vi "Autonomous Independent.vi"() -> ()   [LabVIEW 2016]
doc: "This VI is called when autonomous begins, and will automatically be terminated when autonomous ends. You can carry out timed or sensor driven robot movement independently without needing to return to the caller."
uses:
  <vilib>/Rock Robotics/WPI/ThirdParty/CanMotor/TalonSRX/WPI_CANTalonSRX_APIFeedbackSelect.ctl
  <vilib>/Rock Robotics/WPI/ThirdParty/CanMotor/TalonSRX/WPI_CANTalonSRX_Params.ctl
  <vilib>/Rock Robotics/WPI/ThirdParty/CanMotor/TalonSRX/WPI_CANTalonSRX_APIControlMode.ctl
  <vilib>/Rock Robotics/WPI/Utilities/WPI_GetSetVariantRefNum.vi
  <vilib>/Rock Robotics/Network Tables/NT Read String.vi
  <vilib>/Rock Robotics/Network Tables/NT Write Numeric Array.vi
  <vilib>/Rock Robotics/WPI/RobotDrive/WPI_RobotDriveArcadeDrive_Standard(NoSaturation).vi
  Robot Global Data.vi
panel:
  out "Distance":dbl
  out "Current":dbl
  out "CURRENT":dbl
  out "Distance 5":dbl
  out "Distance 4":dbl
  out "Distance 3":dbl
  out "RIGHT SIDE":dbl
  out "Encoder Position 4":dbl
  out "Encoder Position 3":dbl
  out "Encoder Position":dbl
  out "Encoder Position 2":dbl
  # "Be sure to right-click and choose Data Operations>>Make Current Value default if you want to save the array values with the VI"
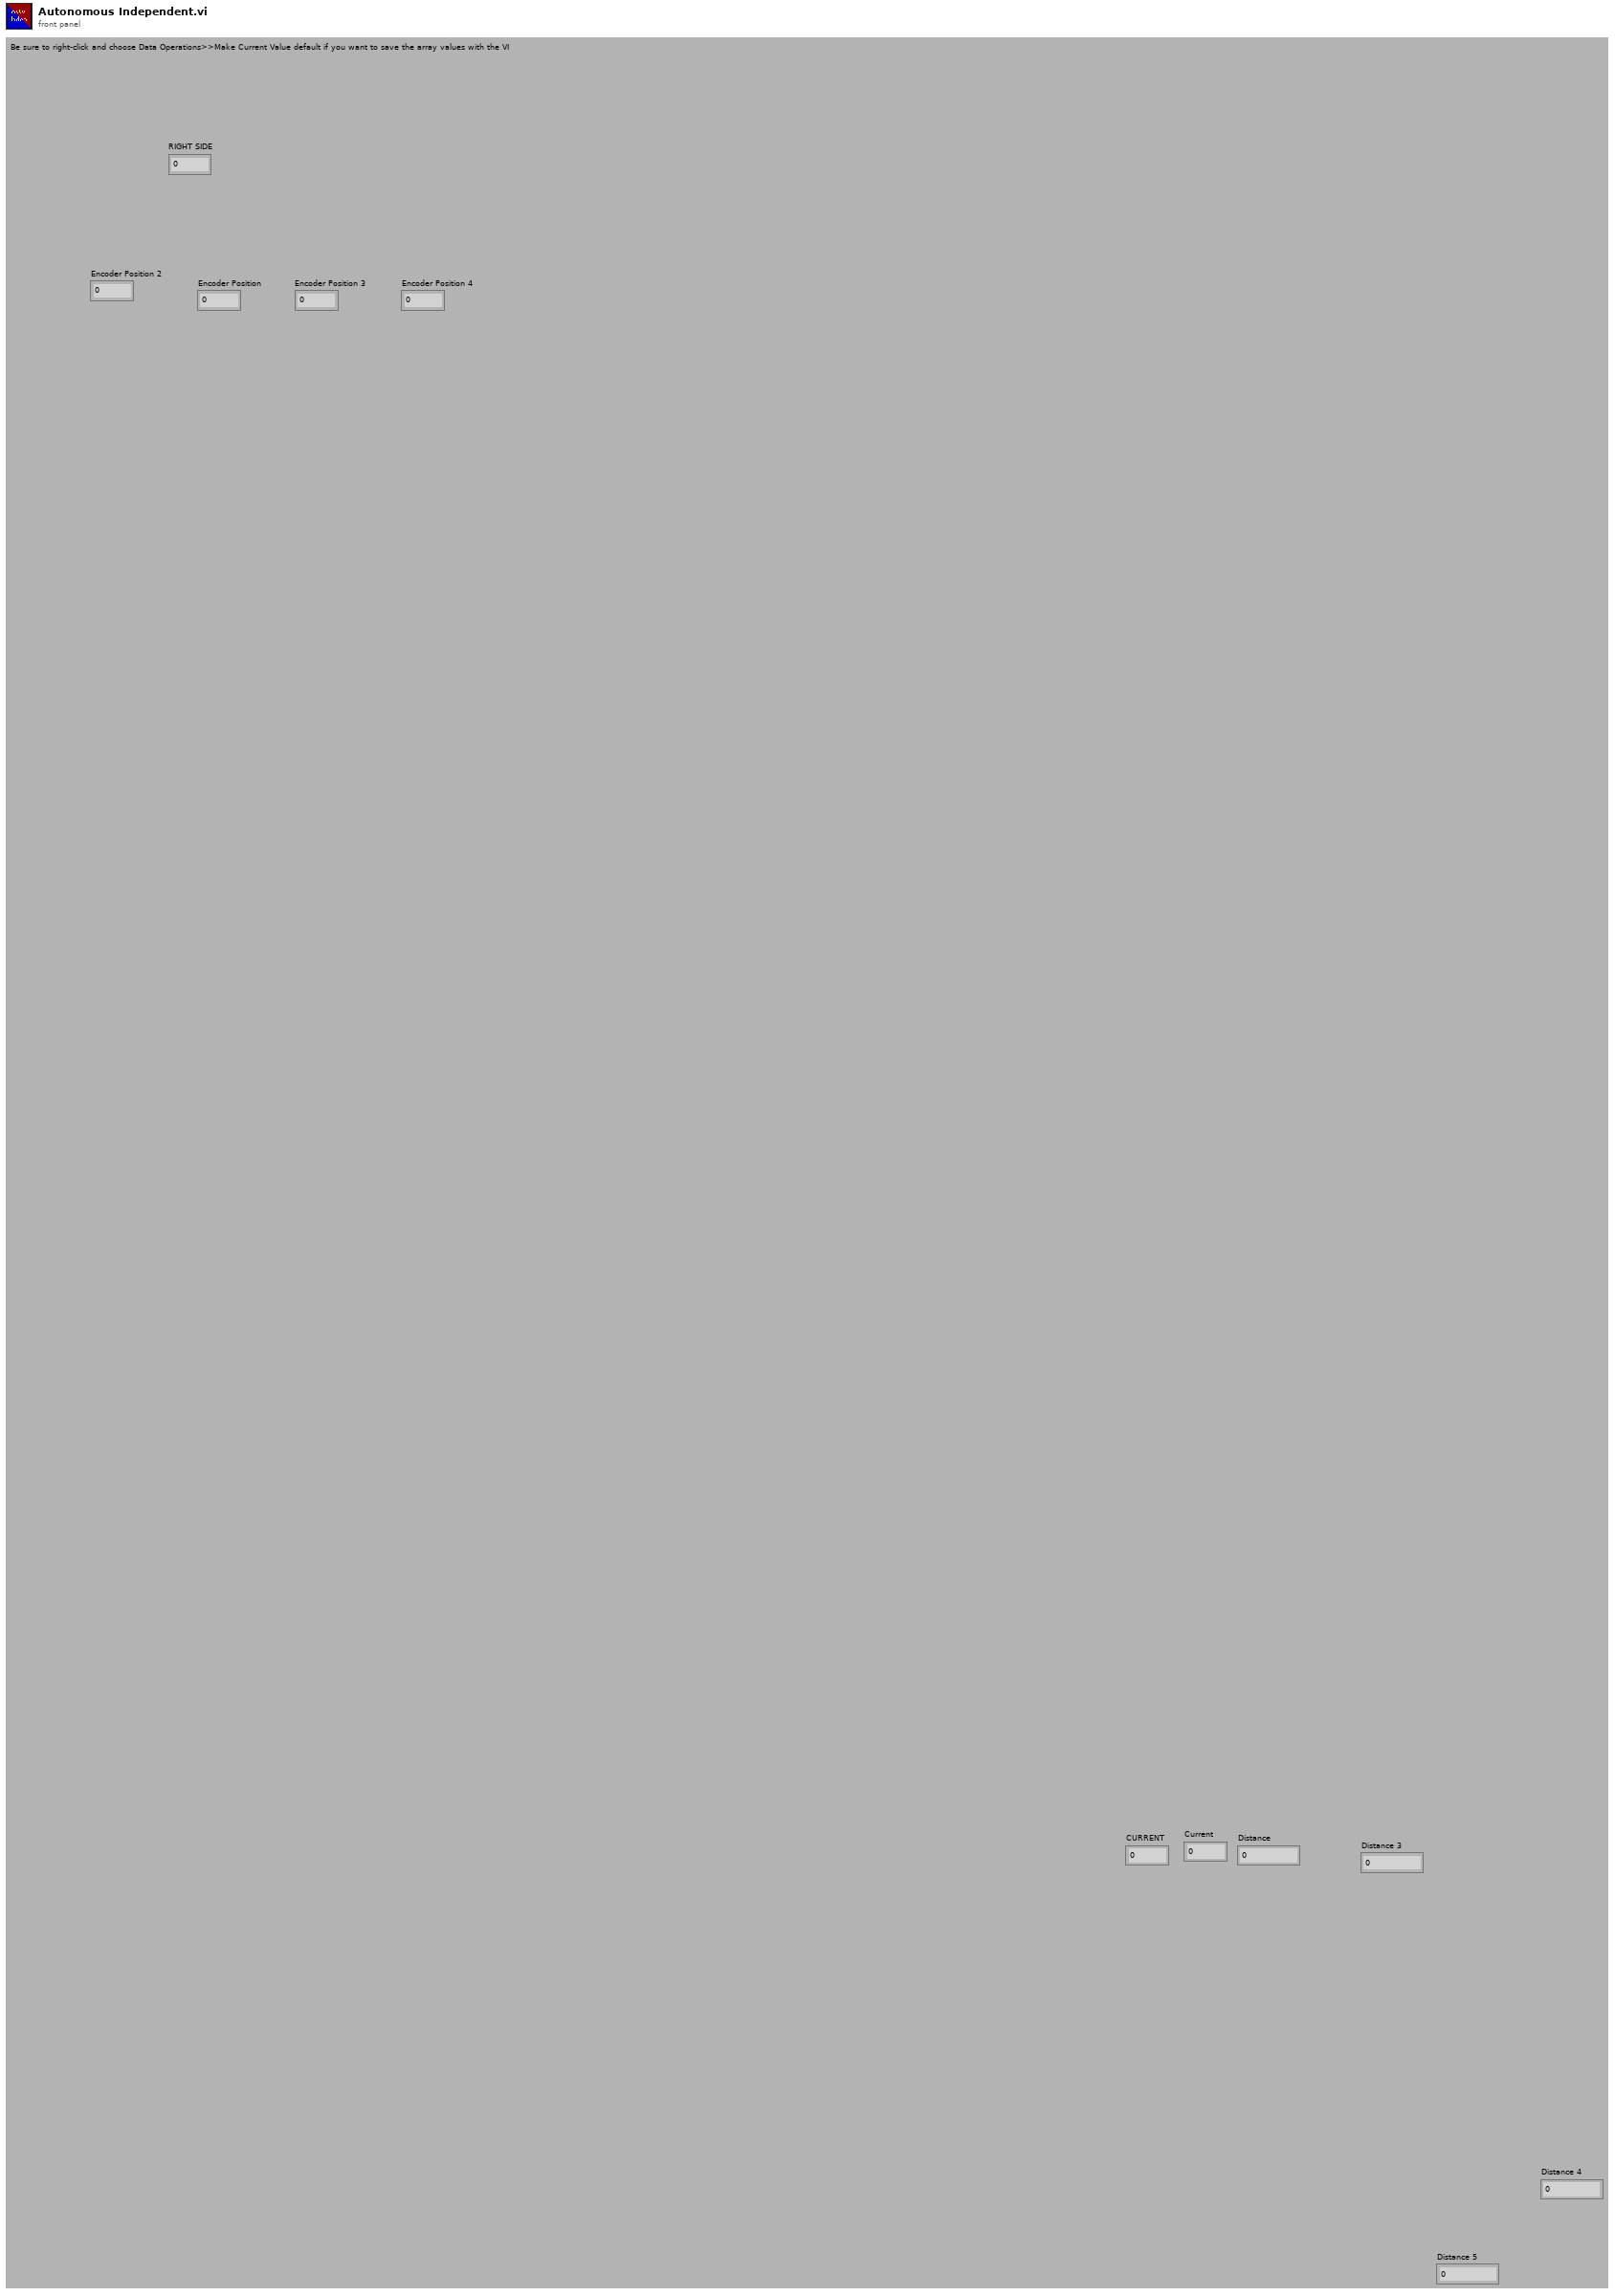
[diagram p1: front panel]
types:
  T1 = typedef "WPI_JoystickDevRef.ctl" = cluster{"Device":T2}
  T2 = typedef "WPI_JoystickDeviceEnum.ctl" = enum16{"USB 0", "USB 1", "USB 2", "USB 3", "USB 4", "USB 5"}
  T3 = typedef "WPI_EncoderDevRef.ctl" = cluster{"DevStatus":errorcluster, "EncoderIndex":T4, "CounterIndex":T5, "DistancePerCount":dbl, "Decoding Type":T6}
  T4 = typedef "FPGA_EncoderIdx.ctl" = enum8{"Enc 0", "Enc 1", "Enc 2", "Enc 3", "Enc 4", "Enc 5", "Enc 6", "Enc 7", "Invalid"}
  T5 = typedef "FPGA_CounterCtrSystemIndex.ctl" = enum8{"Ctr 0", "Ctr 1", "Ctr 2", "Ctr 3", "Ctr 4", "Ctr 5", "Ctr 6", "Ctr 7", "Invalid"}
  T6 = typedef "WPI_EncoderType.ctl" = enum16{"1x", "2x", "4x"}
  T7 = typedef "WPI_MotorControlDeviceRef.ctl" = cluster{"DeviceStatus":errorcluster, "Type":T8, "PWM":cluster{"PWM Channel":T9, "DeadBand":T10}, "CAN":cluster{"Device Number":u8, "SetOutput VI Ref":variant, "GetOutput VI Ref":variant, "Enable VI Ref":variant, "Disable VI Ref":variant, "Data":variant}, "Invert":bool}
  T8 = typedef "WPI_MotorControlType.ctl" = enum16{"PWM", "CAN"}
  T9 = typedef "FPGA_DIOPWMChannel.ctl" = enum8{"PWM 0", "PWM 1", "PWM 2", "PWM 3", "PWM 4", "PWM 5", "PWM 6", "PWM 7", "PWM 8", "PWM 9", "PWM MXP 0", "PWM MXP 1", "PWM MXP 2", "PWM MXP 3", "PWM MXP 4", "PWM MXP 5", "PWM MXP 6", "PWM MXP 7", "PWM MXP 8", "PWM MXP 9", "Invalid"}
  T10 = typedef "WPI_PWMDeadband.ctl" = cluster{"Name":string, "maxPositivePwm":i32, "minPositivePwm":i32, "centerPwm":i32, "maxNegativePwm":i32, "minNegativePwm":i32, "angularRange":u16}
  T11 = typedef "WPI_RobotDriveDevRef.ctl" = cluster{"DevStatus":errorcluster, "Motors[]":T7[], "Square Inputs":bool, "Max Output":dbl}
  T12 = typedef "WPI_CANTalonSRX_APIFeedbackSelect.ctl" = enum16{"Digital Quadrature Encoder", "Analog Potentiometer", "Analog Encoder", "Count on Quad-A (Rising-Edge)", "Count on Quad-A (Falling-Edge)", "CTR Magnetic Enc (Absolute)", "CTR Magnetic Enc (Relative)", "Pulse Width"}
  T13 = typedef "WPI_CANTalonSRX_APIControlMode.ctl" = enum8{"Percent VBus", "Speed", "Position", "Slave", "Unchanged / Invalid", "Voltage Compensation", "Current", "Motion Profile", "Motion Magic"}
  T14 = typedef "WPI_CANTalonSRX_Params.ctl" = u8
  T15 = typedef "WPI_CANTalonSRX_GlobalStatus.ctl" = cluster{"Applied Throttle":dbl, "Module Enabled":bool, "CAN Error":errorcluster, "Closed Loop Error":dbl, "Forward Limit Switch Closed":bool, "Reverse Limit Switch Closed":bool, "Sensor Position":dbl, "Sensor Velocity":dbl, "Current":dbl, "Sticky Fault - Over Temp":bool, "Sticky Fault - Under Voltage":bool, "Sticky Fault - Forward Limit":bool, "Sticky Fault - Reverse Limit":bool, "Sticky Fault - Forward Soft Limit":bool, "Sticky Fault - Reverse Soft Limit":bool, "Brake is Enabled":bool, "Encoder Position":dbl, "Encoder Velocity":dbl, "Encoder Index Count":dbl, "Encoder A Pin State":bool, "Encoder B Pin State":bool, "Encoder Index Pin State":bool, "Analog In":dbl, "Analog In Velocity":dbl, "Temperature (C)":dbl, "Battery Voltage":dbl, "Control 5 Is Supported":bool, "Current Profile Slot Select":dbl, "Pos Div 8":bool, "Vel Div 4":bool, "Pulse Width Position":i32, "Pulse Width Velocity":i32, "Pulse Width Rise To Rise (us)":i32, "Pulse Width Rise To Fall (us)":i32, "Mot Prof Active Is Under Run":bool, "Mot Prof Active Has Under Run":bool, "Mot Prof Active Is Last":bool, "Mot Prof Active Velocity Only":bool, "Mot Prof Active Is Valid":bool, "Mot Prof Buffer Is Full":bool, "Mot Prof Active Profile Slot Select":i32, "Mot Prof NextID":i32, "Mot Prof Count":i32, "Mot Prof Active Velocity":dbl, "Mot Prof Active Position":dbl, "Mot Prof Output Enable":i32, "UsageFrame":u32}
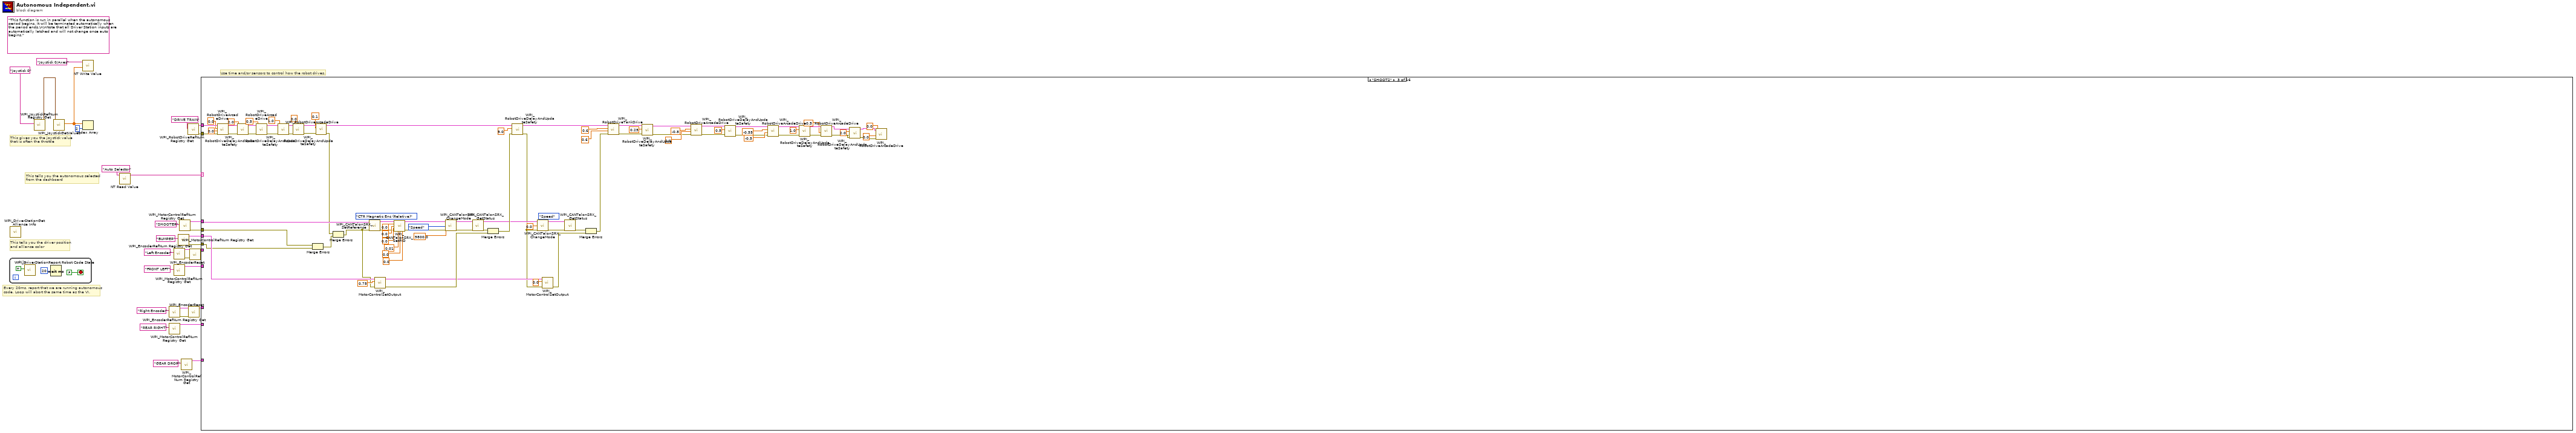
[diagram p0: block diagram]
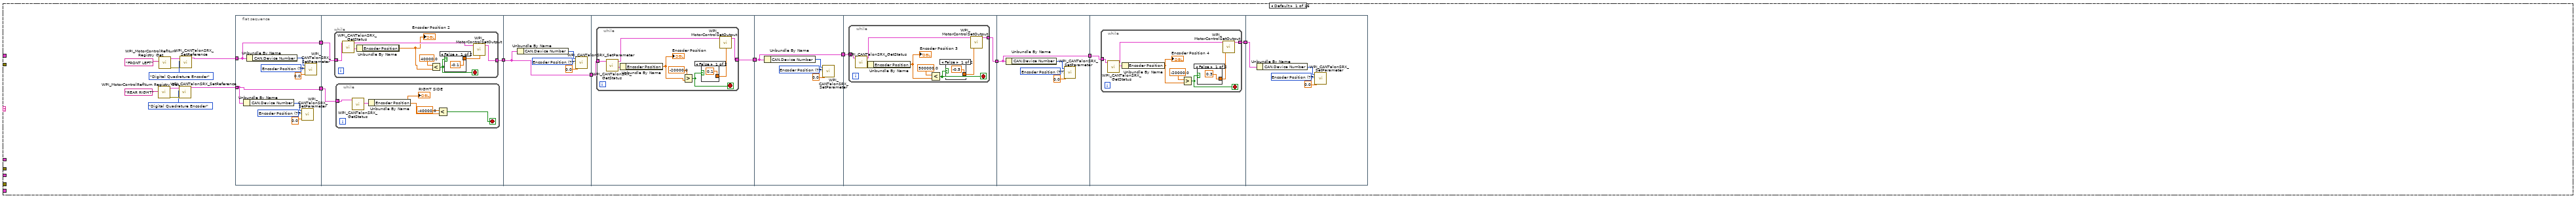
[diagram p2: hidden frame]
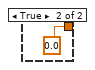
[diagram p3: hidden frame]
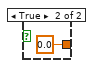
[diagram p4: hidden frame]
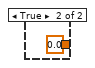
[diagram p5: hidden frame]
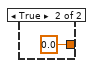
[diagram p6: hidden frame]
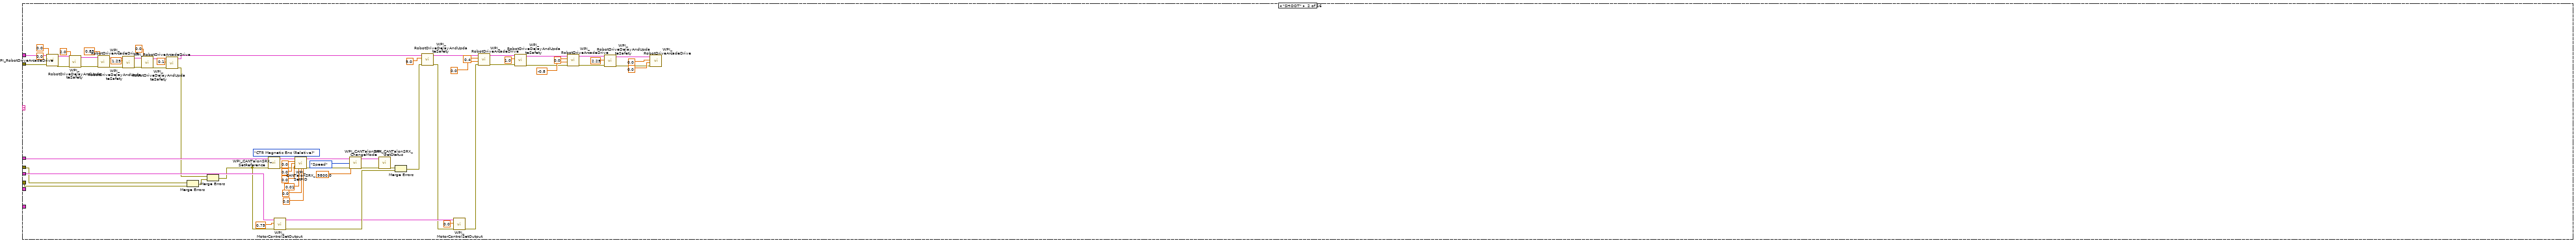
[diagram p7: hidden frame]
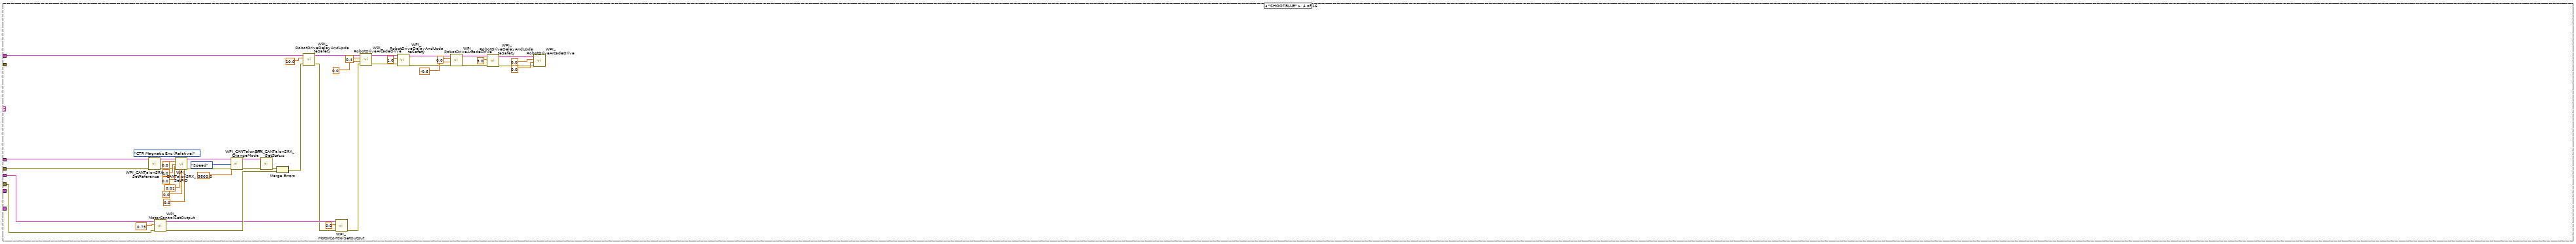
[diagram p8: hidden frame]
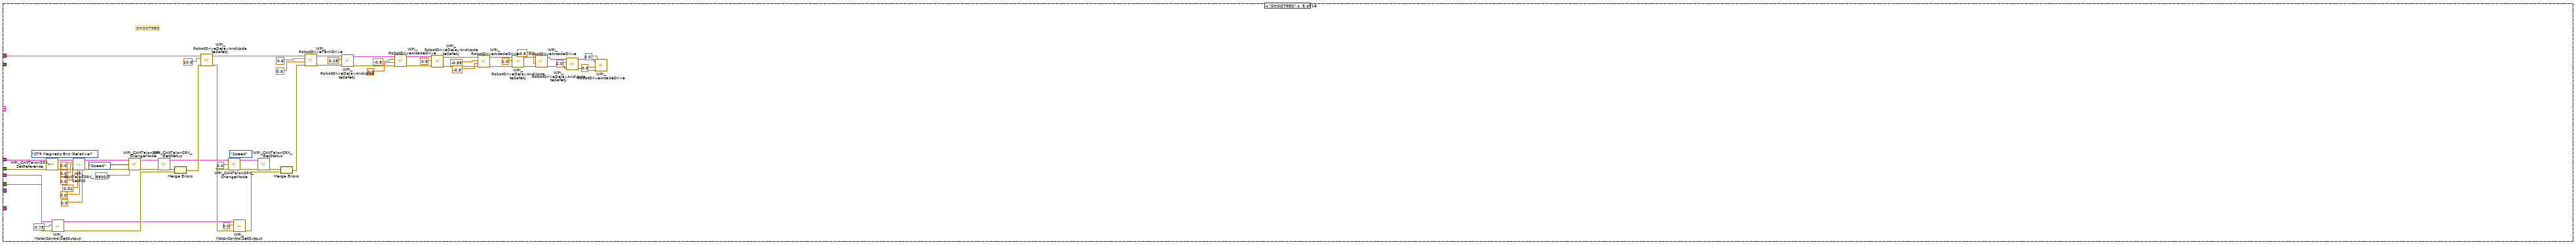
[diagram p9: hidden frame]
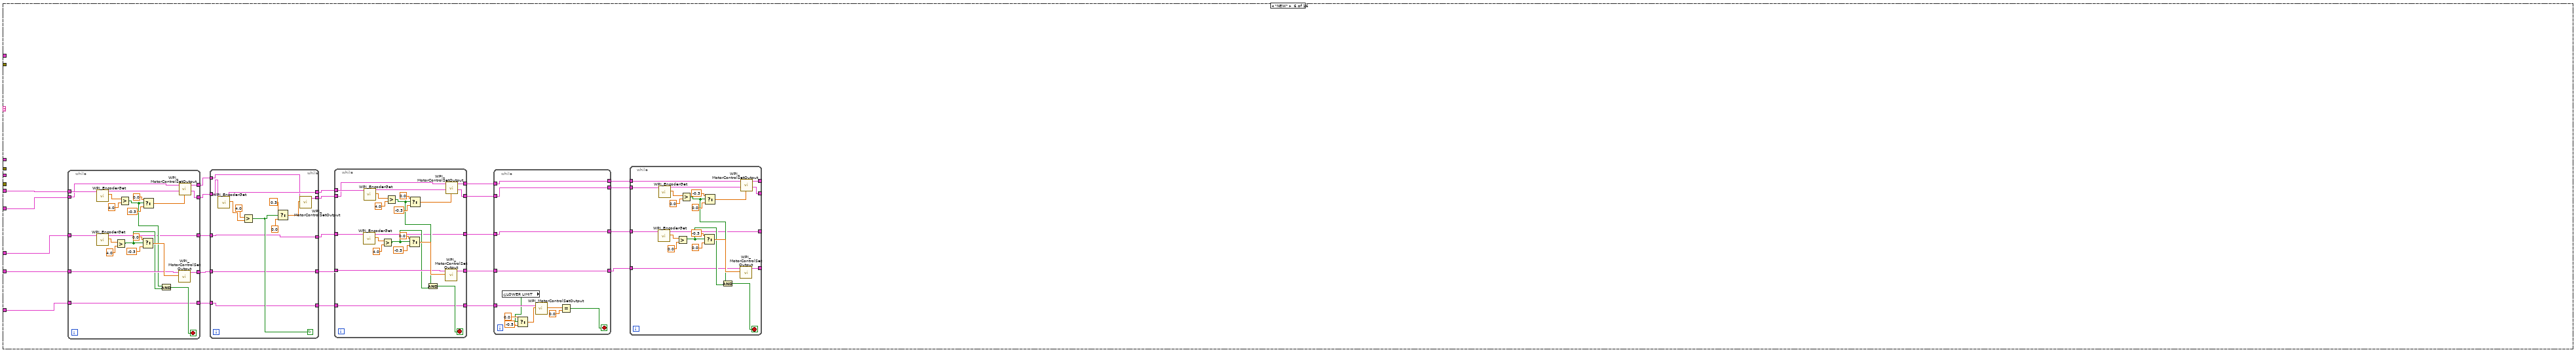
[diagram p10: hidden frame]
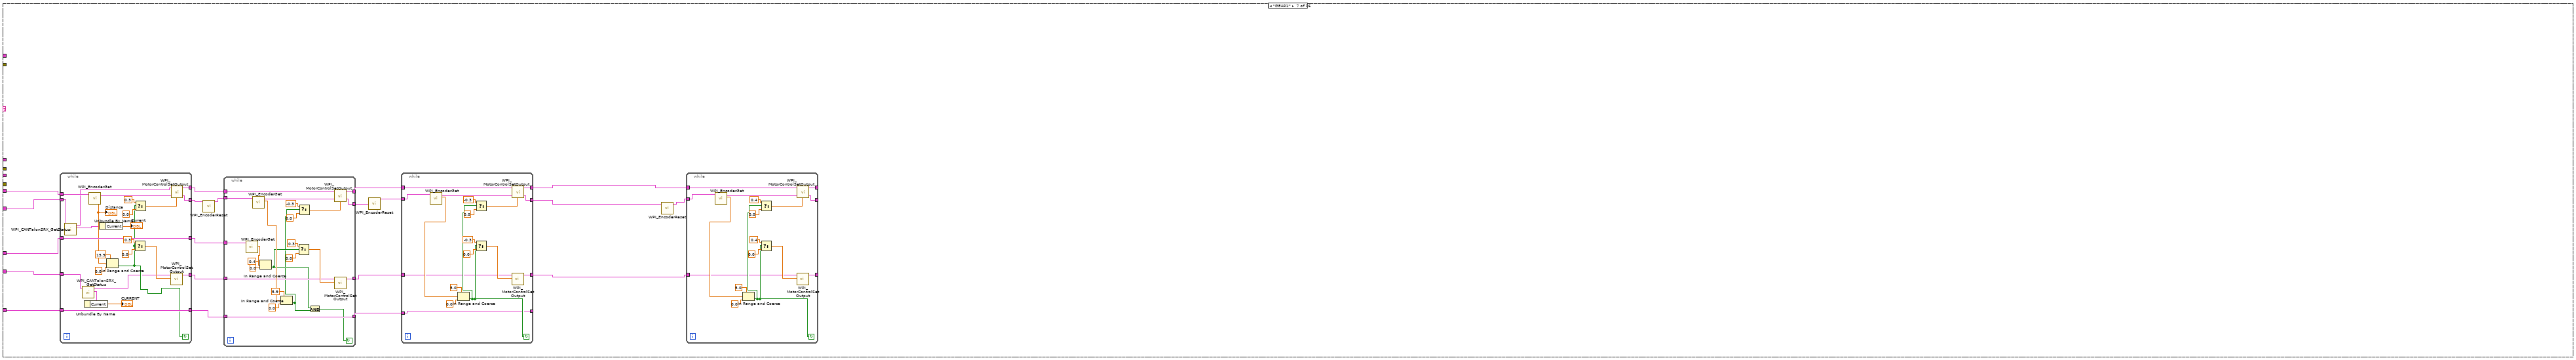
[diagram p11: hidden frame]
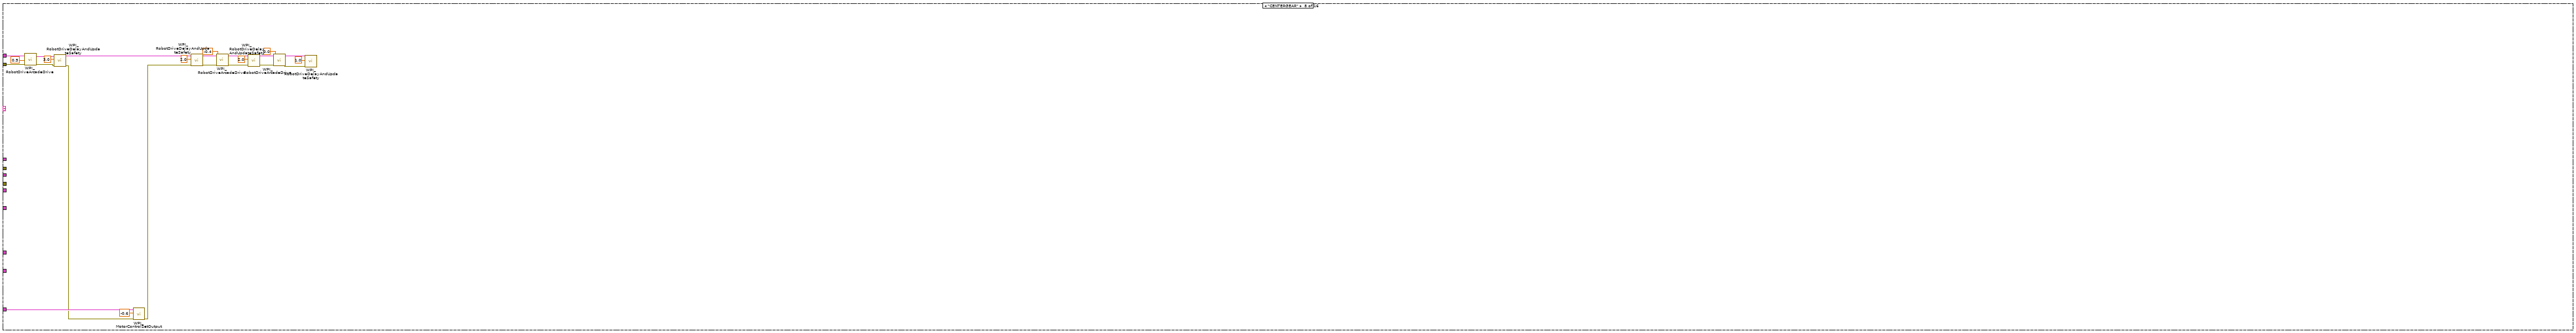
[diagram p12: hidden frame]
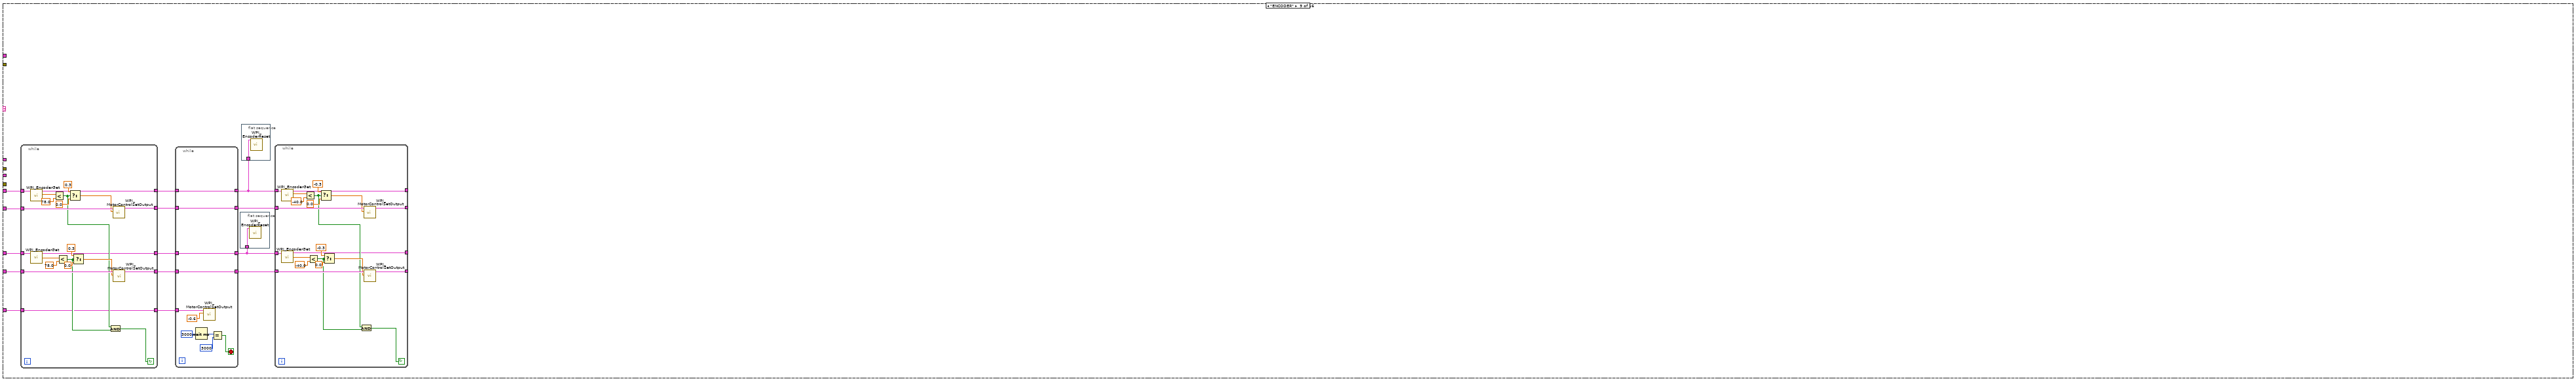
[diagram p13: hidden frame]
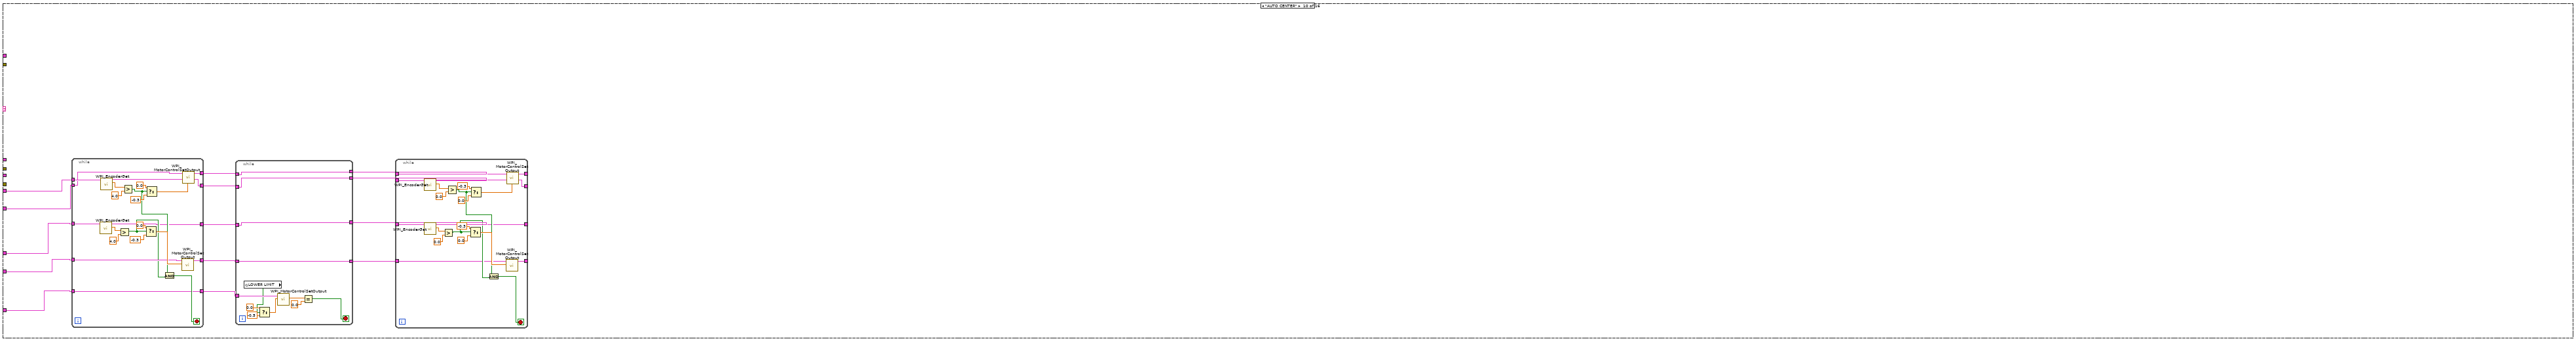
[diagram p14: hidden frame]
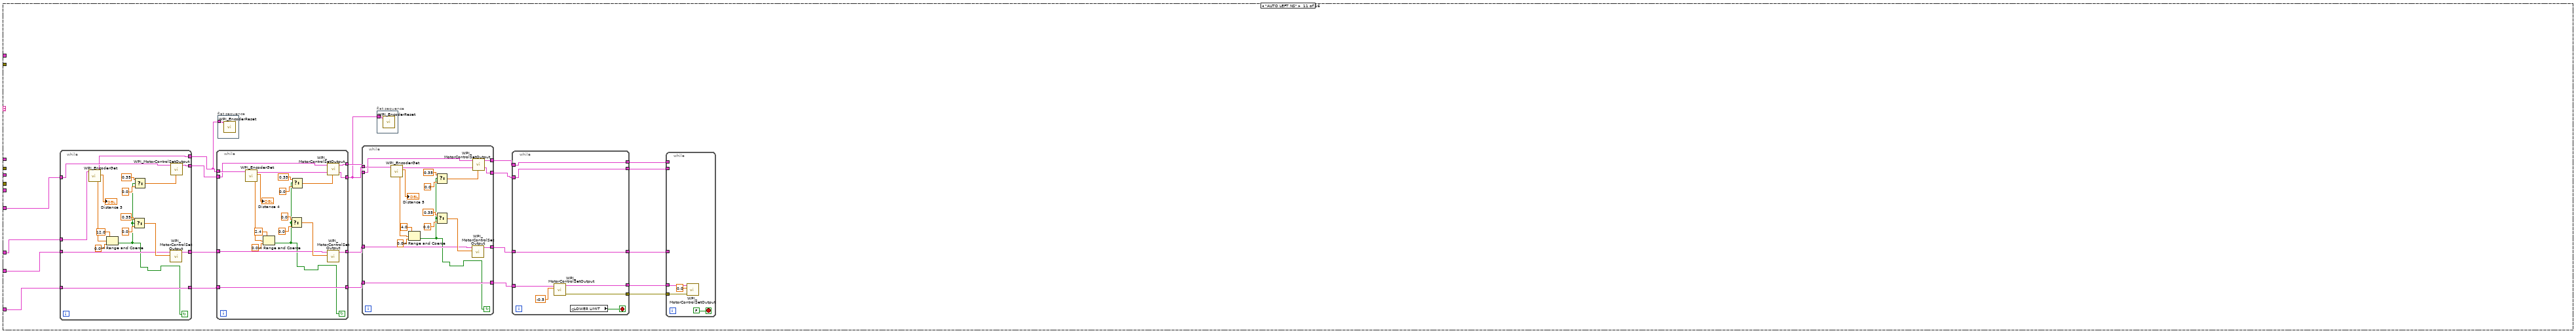
[diagram p15: hidden frame]
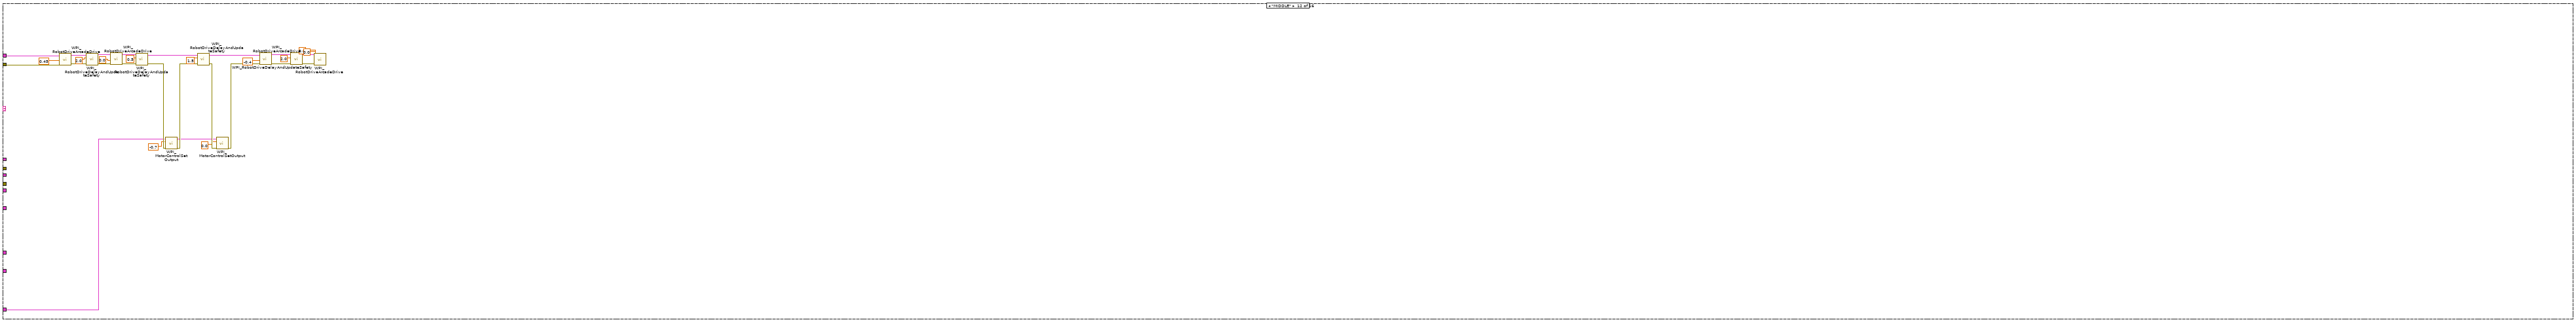
[diagram p16: hidden frame]
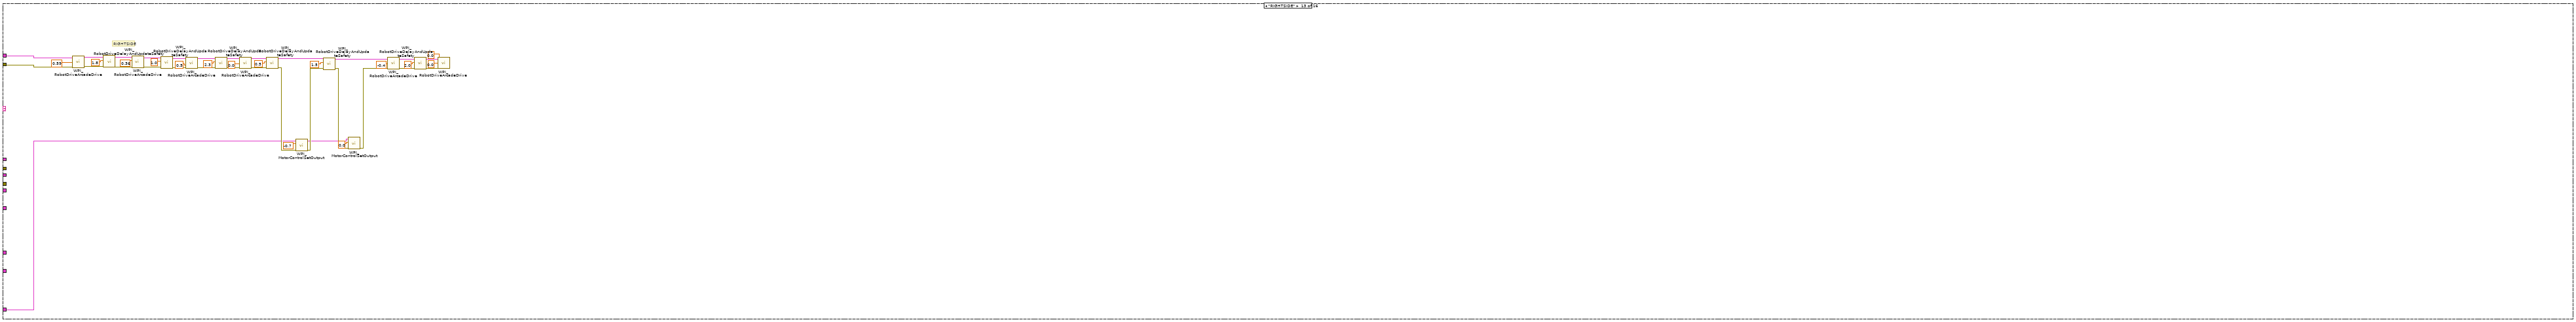
[diagram p17: hidden frame]
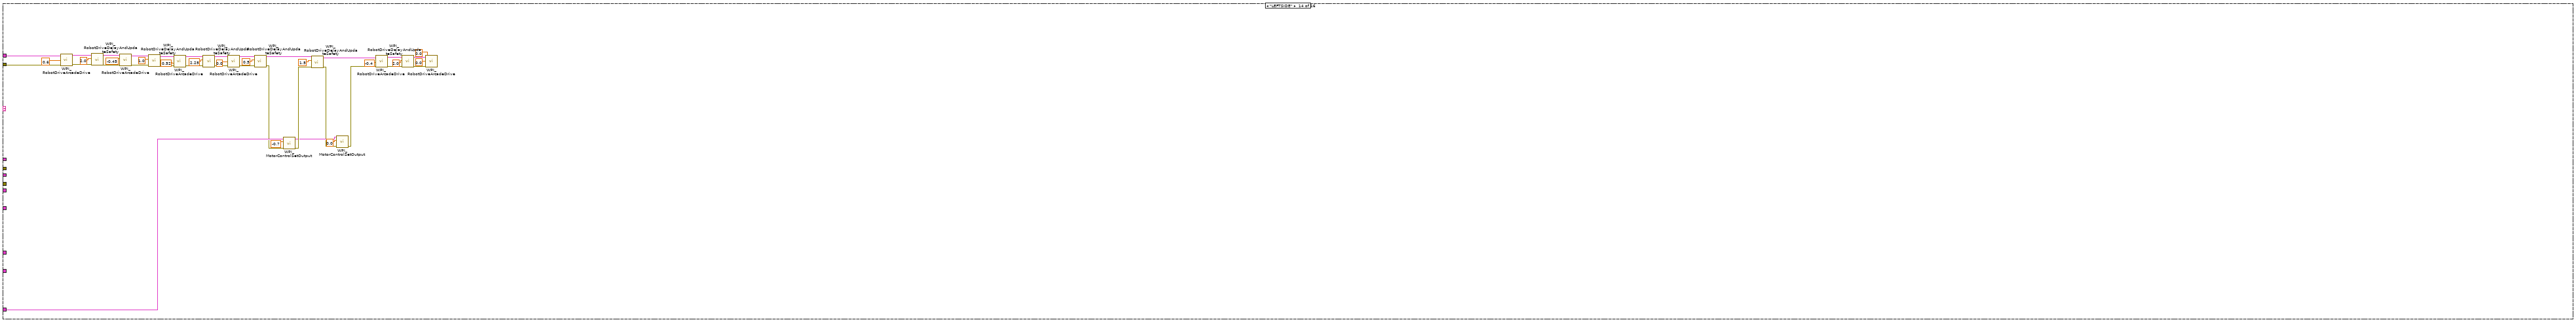
[diagram p18: hidden frame]
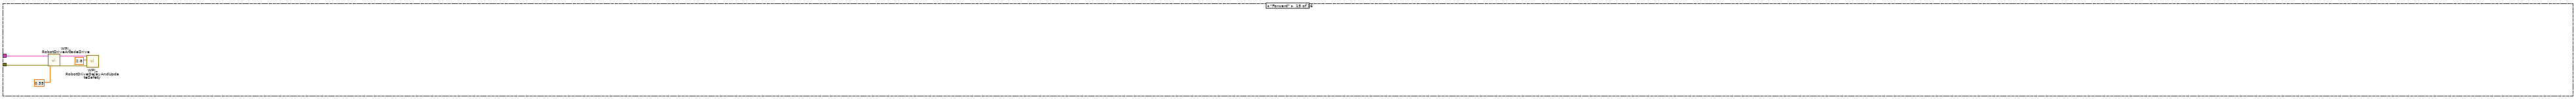
[diagram p19: hidden frame]
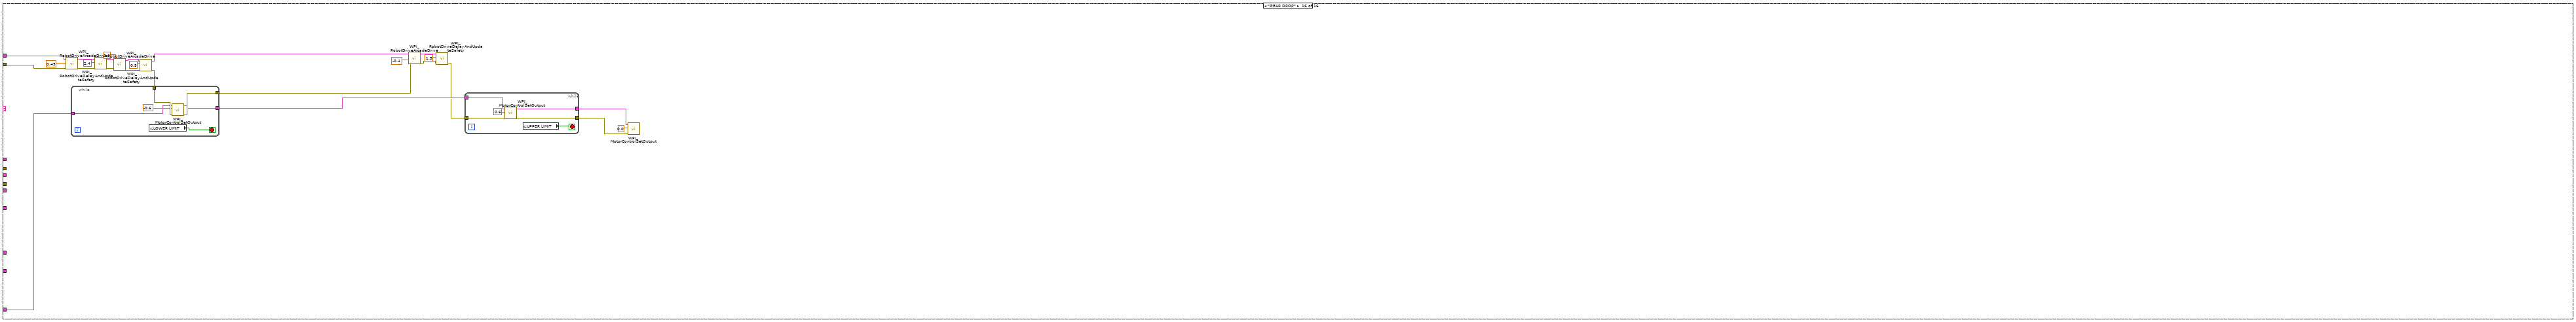
[diagram p20: hidden frame]
diagram:
  (unwired) "This function is run in parallel when the autonomous period begins. It will be terminated automatically when the period ends.\n\nNote that all Driver Station inputs are automatically latched and will not change once auto begins."
  # "Use time and/or sensors to control how the robot drives."
  # "This tells you the autonomous selected\nfrom the dashboard"
  # "Every 20ms, report that we are running autonomous\ncode. Loop will abort the same time as the VI."
  # "This gives you the joystick value\nthat is often the throttle"
  # "This tells you the driver position\nand alliance color"
  n1 = while {
    stop <- FALSE stop-if-true
    n2 = call <vilib>:"WPI_DriverStationReport Robot Code State.vi"("Autonomous"=TRUE) -> ()  [unwired: 10 in, 1 out]
    n3 = Wait (ms)(milliseconds to wait=u32 20) -> ()  [unwired: 1 out]
  }
  n4 = call <vilib>:"WPI_DriverStationGet Alliance Info.vi"() -> ()  [unwired: 12 out]
  n5 = call <vilib>:"WPI_JoystickRefNum Registry Get.vi"("refnum name"="Joystick 0") -> ("JoystickDevRef"=w29:T1)  [unwired: 1 in, 9 out]
  n6 = call <vilib>:"WPI_JoystickGetValues.vi"("JoystickDevRef"=w29) -> ("Axes"=w25:dbl[])  [unwired: 6 in, 4 out]
  n7 = call-poly <vilib>:"NT Write Value.vi"("Numeric Array"=w25, "Name"="Joystick 0/Axes") -> ()  [unwired: 9 in, 1 out]
  n8 = Index Array(array=w25, index=2) -> ()  [unwired: 1 out]
  n9 = call-poly <vilib>:"NT Read Value.vi"("Name"="Auto Selector") -> ("String"=w26:string)  [unwired: 9 in, 1 out]
  n10 = call <vilib>:"WPI_EncoderRefNum Registry Get.vi"("refnum name"="Right Encoder") -> ("error out"=w6:errorcluster, "EncoderDevRef"=w5:T3)  [unwired: 9 in]
  n11 = call <vilib>:"WPI_MotorControlRefNum Registry Get.vi"("refnum name"="REAR RIGHT") -> ("MotorControlDevRef"=w7:T7)  [unwired: 9 in, 1 out]
  n12 = call <vilib>:"WPI_EncoderRefNum Registry Get.vi"("refnum name"="Left Encoder") -> ("error out"=w3:errorcluster, "EncoderDevRef"=w2:T3)  [unwired: 9 in]
  n13 = call <vilib>:"WPI_MotorControlRefNum Registry Get.vi"("refnum name"="FRONT LEFT") -> ("MotorControlDevRef"=w10:T7)  [unwired: 9 in, 1 out]
  n14 = call <vilib>:"WPI_MotorControlRefNum Registry Get.vi"("refnum name"="BUMPER") -> ("error out"=w14:errorcluster, "MotorControlDevRef"=w15:T7)  [unwired: 9 in]
  n15 = call <vilib>:"WPI_MotorControlRefNum Registry Get.vi"("refnum name"="SHOOTER") -> ("error out"=w16:errorcluster, "MotorControlDevRef"=w17:T7)  [unwired: 9 in]
  n16 = call <vilib>:"WPI_MotorControlRefNum Registry Get.vi"("refnum name"="GEAR DROP") -> ("MotorControlDevRef"=w19:T7)  [unwired: 9 in, 1 out]
  n17 = call <vilib>:"WPI_RobotDriveRefNum Registry Get.vi"("refnum name"="DRIVE TRAIN") -> ("error out"=w21:errorcluster, "RobotDriveDevRef"=w22:T11)  [unwired: 9 in]
  n18 = call <vilib>:"WPI_EncoderReset.vi"("error in (no error)"=w6, "EncoderDevRef"=w5) -> ("EncoderDevRef"=w4:T3)  [unwired: 8 in, 1 out]
  n19 = call <vilib>:"WPI_EncoderReset.vi"("error in (no error)"=w3, "EncoderDevRef"=w2) -> ("EncoderDevRef"=w1:T3)  [unwired: 8 in, 1 out]
  n20 = case shown="\"SHOOT2\"" w26 {
    tunnel: w22 -> [_ w156 w224 w291 w380 _ _ w636 _ _ _ w891 w894 w977 w983 w1008]
    tunnel: w21 -> [_ w155 w225 _ _ _ _ w635 _ _ _ w890 w893 w976 w982 w1007]
    tunnel: w19 -> [_ _ _ _ _ w406 w528 w630 w646 w715 w793 w878 w892 w953 _ w988]
    tunnel: w17 -> [_ w186 w205 w287 w386 _ _ _ _ _ _ _ _ _ _ _]
    tunnel: w16 -> [_ w143 w203 w288 w385 _ _ _ _ _ _ _ _ _ _ _]
    tunnel: w15 -> [_ w173 w204 w290 w373 _ _ _ _ _ _ _ _ _ _ _]
    tunnel: w14 -> [_ w142 w202 w289 w372 _ _ _ _ _ _ _ _ _ _ _]
    tunnel: w1 -> [_ _ _ _ _ w420 w531 _ w650 w719 _ _ _ _ _ _]
    tunnel: w10 -> [_ _ _ _ _ w419 w532 _ w649 w718 w795 _ _ _ _ _]
    tunnel: w7 -> [_ _ _ _ _ w417 w529 _ w647 w716 w794 _ _ _ _ _]
    tunnel: w4 -> [_ _ _ _ _ w418 w530 _ w648 w717 w775 _ _ _ _ _]
    frame Default {
      n21 = call <vilib>:"WPI_MotorControlRefNum Registry Get.vi"("refnum name"="REAR RIGHT") -> ("error out"=w38:errorcluster, "MotorControlDevRef"=w37:T7)  [unwired: 9 in]
      n22 = call <vilib>:"WPI_MotorControlRefNum Registry Get.vi"("refnum name"="FRONT LEFT") -> ("error out"=w50:errorcluster, "MotorControlDevRef"=w51:T7)  [unwired: 9 in]
      n23 = call <vilib>:"WPI_CANTalonSRX_SetReference.vi"("error in (no error)"=w38, "Feedback Reference"=WPI_CANTalonSRX_APIFeedbackSelect."Digital Quadrature Encoder", "CAN Talon SRX Ref"=w37) -> ("CAN Talon SRX Ref"=w35:T7)  [unwired: 7 in, 1 out]
      n24 = call <vilib>:"WPI_CANTalonSRX_SetReference.vi"("error in (no error)"=w50, "Feedback Reference"=WPI_CANTalonSRX_APIFeedbackSelect."Digital Quadrature Encoder", "CAN Talon SRX Ref"=w51) -> ("CAN Talon SRX Ref"=w46:T7)  [unwired: 7 in, 1 out]
      n25 = flat-sequence {
        tunnel: w46 -> [w57]
        tunnel: [w57] -> w45
        tunnel: w35 -> [w53]
        tunnel: [w53] -> w34
        tunnel: [w62] -> w48
        tunnel: w45 -> [w63]
        tunnel: w34 -> [w61]
        tunnel: w48 -> [w79]
        tunnel: [w79] -> w47
        tunnel: w47 -> [w84]
        tunnel: [w83] -> w44
        tunnel: w44 -> [w95]
        tunnel: [w95] -> w43
        tunnel: w43 -> [w100]
        tunnel: [w99] -> w42
        tunnel: w42 -> [w111]
        tunnel: [w111] -> w41
        tunnel: w41 -> [w116]
        tunnel: [w115] -> w40
        tunnel: w40 -> [w127]
        frame #0 {
          w55 = T14 77 items=["Slot 0 - P"=1, "Slot 0 - I"=2, "Slot 0 - D"=3, "Slot 0 - F"=4, "Slot 0 - I Zone"=5, "Slot 0 - Ramp Rate"=6, "Slot 1 - P"=11, "Slot 1 - I"=12, "Slot 1 - D"=13, "Slot 1 - F"=14, "Slot 1 - I Zone"=15, "Slot 1 - Ramp Rate"=16, "Soft Limit - Forward"=21, "Soft Limit - Reverse"=22, "Soft Limit - Forward Enable"=23, "Soft Limit - Reverse Enable"=24, "On Boot - Brake Mode"=31, "On Boot - Limit Normally Closed - Forward"=32, "On Boot - Limit Normally Closed - Reverse"=33, "On Boot - Limit Disabled - Forward"=34, "On Boot - Limit Disabled - Reverse"=35, "Fault - Over Temp"=41, "Fault - Under Voltage"=42, "Fault - Forward Limit"=43, "Fault - Reverse Limit"=44, "Fault - Hardware Failure"=45, "Fault - Forward Soft Limit"=46, "Fault - Reverse Soft Limit"=47, "Sticky Fault - Over Temp"=48, "Sticky Fault - Under Voltage"=49, "Sticky Fault - Forward Limit"=50, "Sticky Fault - Reverse Limit"=51, "Sticky Fault - Forward Soft Limit"=52, "Sticky Fault - Reverse Soft Limit"=53, "Applied Throttle"=61, "Closed-Loop Error"=62, "Select Feedback Device"=63, "Reverse Closed-Loop Output"=64, "Mode Select"=65, "Profile Slot Select"=66, "Ramp Throttle"=67, "Reverse Feedback Sensor"=68, "Limit Switch Enabled"=69, "Limit Switch Closed - Forward"=70, "Limit Switch Closed - Reverse"=71, "Sensor Position"=73, "Sensor Velocity"=74, "Current"=75, "Brake is Enabled"=76, "Encoder Position"=77, "Encoder Velocity"=78, "Encoder Index Rise Events"=79, "Encoder A Pin State"=80, "Encoder B Pin State"=81, "Encoder Index Pin State"=82, "Analog In with Overflow"=83, "Analog In Velocity"=84, "Temperature"=85, "Battery Voltage"=86, "Reset Count"=87, "Reset Flags"=88, "Firmware Version"=89, "Settings Changed"=90, "Quad Filter Enable"=91, "Ignore Disable Broadcast"=92, "I Accumulator"=93, "Status 1 Frame Rate Ms"=94, "Status 2 Frame Rate Ms"=95, "Status 3 Frame Rate Ms"=96, "Status 4 Frame Rate Ms"=97, "Status 6 Frame Rate Ms"=98, "Status 7 Frame Rate Ms"=99, "Enable Index Pin Clear Position"=100, "Peak Positive Output"=104, "Nominal Positive Output"=105, "Peak Negative Output"=106, "Nominal Negative Output"=107, "Quad Index Pin Polarity"=108, "Status 8 Frame Rate Ms"=109, "Allow Position Overflow"=110, "Slot 0 - Allowable Closed-Loop Error"=111, "Number Potentiometer Turns"=112, "Encoder Codes Per Rev"=113, "Pulse Width Decoded Position"=114, "Analog Position"=115, "Voltage Compensation Rate (V/s)"=116, "Slot 1 - Allowable Closed-Loop Error"=117, "Motion Profile Has Underrun Err"=119, "Reserved 120"=120, "Legacy Control Mode"=121, "Motion Magic Acceleration"=122, "Motion Magic Cruise Velocity"=123, "Status 10 Frame Rate"=124, "Current Limit Threshold"=125, "CustomParam0"=137, "CustomParam1"=138, "PersStorageSaving"=139, "ClearPositionOnLimitF"=144, "ClearPositionOnLimitR"=145, "NominalBatteryVoltage"=146, "SampleVelocityPeriod"=147, "SampleVelocityWindow"=148] ("Parameter")
          w59 = T14 77 items=["Slot 0 - P"=1, "Slot 0 - I"=2, "Slot 0 - D"=3, "Slot 0 - F"=4, "Slot 0 - I Zone"=5, "Slot 0 - Ramp Rate"=6, "Slot 1 - P"=11, "Slot 1 - I"=12, "Slot 1 - D"=13, "Slot 1 - F"=14, "Slot 1 - I Zone"=15, "Slot 1 - Ramp Rate"=16, "Soft Limit - Forward"=21, "Soft Limit - Reverse"=22, "Soft Limit - Forward Enable"=23, "Soft Limit - Reverse Enable"=24, "On Boot - Brake Mode"=31, "On Boot - Limit Normally Closed - Forward"=32, "On Boot - Limit Normally Closed - Reverse"=33, "On Boot - Limit Disabled - Forward"=34, "On Boot - Limit Disabled - Reverse"=35, "Fault - Over Temp"=41, "Fault - Under Voltage"=42, "Fault - Forward Limit"=43, "Fault - Reverse Limit"=44, "Fault - Hardware Failure"=45, "Fault - Forward Soft Limit"=46, "Fault - Reverse Soft Limit"=47, "Sticky Fault - Over Temp"=48, "Sticky Fault - Under Voltage"=49, "Sticky Fault - Forward Limit"=50, "Sticky Fault - Reverse Limit"=51, "Sticky Fault - Forward Soft Limit"=52, "Sticky Fault - Reverse Soft Limit"=53, "Applied Throttle"=61, "Closed-Loop Error"=62, "Select Feedback Device"=63, "Reverse Closed-Loop Output"=64, "Mode Select"=65, "Profile Slot Select"=66, "Ramp Throttle"=67, "Reverse Feedback Sensor"=68, "Limit Switch Enabled"=69, "Limit Switch Closed - Forward"=70, "Limit Switch Closed - Reverse"=71, "Sensor Position"=73, "Sensor Velocity"=74, "Current"=75, "Brake is Enabled"=76, "Encoder Position"=77, "Encoder Velocity"=78, "Encoder Index Rise Events"=79, "Encoder A Pin State"=80, "Encoder B Pin State"=81, "Encoder Index Pin State"=82, "Analog In with Overflow"=83, "Analog In Velocity"=84, "Temperature"=85, "Battery Voltage"=86, "Reset Count"=87, "Reset Flags"=88, "Firmware Version"=89, "Settings Changed"=90, "Quad Filter Enable"=91, "Ignore Disable Broadcast"=92, "I Accumulator"=93, "Status 1 Frame Rate Ms"=94, "Status 2 Frame Rate Ms"=95, "Status 3 Frame Rate Ms"=96, "Status 4 Frame Rate Ms"=97, "Status 6 Frame Rate Ms"=98, "Status 7 Frame Rate Ms"=99, "Enable Index Pin Clear Position"=100, "Peak Positive Output"=104, "Nominal Positive Output"=105, "Peak Negative Output"=106, "Nominal Negative Output"=107, "Quad Index Pin Polarity"=108, "Status 8 Frame Rate Ms"=109, "Allow Position Overflow"=110, "Slot 0 - Allowable Closed-Loop Error"=111, "Number Potentiometer Turns"=112, "Encoder Codes Per Rev"=113, "Pulse Width Decoded Position"=114, "Analog Position"=115, "Voltage Compensation Rate (V/s)"=116, "Slot 1 - Allowable Closed-Loop Error"=117, "Motion Profile Has Underrun Err"=119, "Reserved 120"=120, "Legacy Control Mode"=121, "Motion Magic Acceleration"=122, "Motion Magic Cruise Velocity"=123, "Status 10 Frame Rate"=124, "Current Limit Threshold"=125, "CustomParam0"=137, "CustomParam1"=138, "PersStorageSaving"=139, "ClearPositionOnLimitF"=144, "ClearPositionOnLimitR"=145, "NominalBatteryVoltage"=146, "SampleVelocityPeriod"=147, "SampleVelocityWindow"=148] ("Parameter")
          n26 = Unbundle By Name(w53) -> ("CAN.Device Number"=w54:u8)
          n27 = Unbundle By Name(w57) -> ("CAN.Device Number"=w60:u8)
          n28 = call <vilib>:"WPI_CANTalonSRX_SetParameter.vi"("Value"=0.0, "Parameter"=w55, "Device ID (0)"=w54) -> ()  [unwired: 7 in, 2 out]
          n29 = call <vilib>:"WPI_CANTalonSRX_SetParameter.vi"("Value"=0.0, "Parameter"=w59, "Device ID (0)"=w60) -> ()  [unwired: 7 in, 2 out]
        }
        frame #1 {
          n30 = while {
            tunnel: w63 -> [w70]
            tunnel: [w69] -> w62
            stop <- w73 stop-if-true
            n31 = call <vilib>:"WPI_CANTalonSRX_GetStatus.vi"("CAN Talon SRX Ref"=w70) -> ("Talon SRX Status"=w76:T15, "CAN Talon SRX Ref"=w75:T7)  [unwired: 8 in, 1 out]
            n32 = Unbundle By Name(w76) -> ("Encoder Position"=w72:dbl)
            "Encoder Position 2" <- w72
            n33 = Less?(x=40000.0, y=w72) -> (x < y?=w73:bool)
            n34 = case shown="False" w73 {
              tunnel: [-0.1 ("x") 0.0 ("x")] -> w74
              frame False {
              }
              frame True {
              }
            }
            n35 = call <vilib>:"WPI_MotorControlSetOutput.vi"("Output"=w74, "MotorControlDevRef"=w75) -> ("MotorControlDevRef"=w69:T7)  [unwired: 7 in, 2 out]
          }
          n36 = while {
            tunnel: w61 -> [w68]
            stop <- w65 stop-if-true
            n37 = call <vilib>:"WPI_CANTalonSRX_GetStatus.vi"("CAN Talon SRX Ref"=w68) -> ("Talon SRX Status"=w64:T15)  [unwired: 8 in, 2 out]
            n38 = Unbundle By Name(w64) -> ("Encoder Position"=w67:dbl)
            "RIGHT SIDE" <- w67
            n39 = Less?(x=-40000.0, y=w67) -> (x < y?=w65:bool)
          }
        }
        frame #2 {
          w81 = T14 77 items=["Slot 0 - P"=1, "Slot 0 - I"=2, "Slot 0 - D"=3, "Slot 0 - F"=4, "Slot 0 - I Zone"=5, "Slot 0 - Ramp Rate"=6, "Slot 1 - P"=11, "Slot 1 - I"=12, "Slot 1 - D"=13, "Slot 1 - F"=14, "Slot 1 - I Zone"=15, "Slot 1 - Ramp Rate"=16, "Soft Limit - Forward"=21, "Soft Limit - Reverse"=22, "Soft Limit - Forward Enable"=23, "Soft Limit - Reverse Enable"=24, "On Boot - Brake Mode"=31, "On Boot - Limit Normally Closed - Forward"=32, "On Boot - Limit Normally Closed - Reverse"=33, "On Boot - Limit Disabled - Forward"=34, "On Boot - Limit Disabled - Reverse"=35, "Fault - Over Temp"=41, "Fault - Under Voltage"=42, "Fault - Forward Limit"=43, "Fault - Reverse Limit"=44, "Fault - Hardware Failure"=45, "Fault - Forward Soft Limit"=46, "Fault - Reverse Soft Limit"=47, "Sticky Fault - Over Temp"=48, "Sticky Fault - Under Voltage"=49, "Sticky Fault - Forward Limit"=50, "Sticky Fault - Reverse Limit"=51, "Sticky Fault - Forward Soft Limit"=52, "Sticky Fault - Reverse Soft Limit"=53, "Applied Throttle"=61, "Closed-Loop Error"=62, "Select Feedback Device"=63, "Reverse Closed-Loop Output"=64, "Mode Select"=65, "Profile Slot Select"=66, "Ramp Throttle"=67, "Reverse Feedback Sensor"=68, "Limit Switch Enabled"=69, "Limit Switch Closed - Forward"=70, "Limit Switch Closed - Reverse"=71, "Sensor Position"=73, "Sensor Velocity"=74, "Current"=75, "Brake is Enabled"=76, "Encoder Position"=77, "Encoder Velocity"=78, "Encoder Index Rise Events"=79, "Encoder A Pin State"=80, "Encoder B Pin State"=81, "Encoder Index Pin State"=82, "Analog In with Overflow"=83, "Analog In Velocity"=84, "Temperature"=85, "Battery Voltage"=86, "Reset Count"=87, "Reset Flags"=88, "Firmware Version"=89, "Settings Changed"=90, "Quad Filter Enable"=91, "Ignore Disable Broadcast"=92, "I Accumulator"=93, "Status 1 Frame Rate Ms"=94, "Status 2 Frame Rate Ms"=95, "Status 3 Frame Rate Ms"=96, "Status 4 Frame Rate Ms"=97, "Status 6 Frame Rate Ms"=98, "Status 7 Frame Rate Ms"=99, "Enable Index Pin Clear Position"=100, "Peak Positive Output"=104, "Nominal Positive Output"=105, "Peak Negative Output"=106, "Nominal Negative Output"=107, "Quad Index Pin Polarity"=108, "Status 8 Frame Rate Ms"=109, "Allow Position Overflow"=110, "Slot 0 - Allowable Closed-Loop Error"=111, "Number Potentiometer Turns"=112, "Encoder Codes Per Rev"=113, "Pulse Width Decoded Position"=114, "Analog Position"=115, "Voltage Compensation Rate (V/s)"=116, "Slot 1 - Allowable Closed-Loop Error"=117, "Motion Profile Has Underrun Err"=119, "Reserved 120"=120, "Legacy Control Mode"=121, "Motion Magic Acceleration"=122, "Motion Magic Cruise Velocity"=123, "Status 10 Frame Rate"=124, "Current Limit Threshold"=125, "CustomParam0"=137, "CustomParam1"=138, "PersStorageSaving"=139, "ClearPositionOnLimitF"=144, "ClearPositionOnLimitR"=145, "NominalBatteryVoltage"=146, "SampleVelocityPeriod"=147, "SampleVelocityWindow"=148] ("Parameter")
          n40 = Unbundle By Name(w79) -> ("CAN.Device Number"=w82:u8)
          n41 = call <vilib>:"WPI_CANTalonSRX_SetParameter.vi"("Value"=0.0, "Parameter"=w81, "Device ID (0)"=w82) -> ()  [unwired: 7 in, 2 out]
        }
        frame #3 {
          n42 = while {
            tunnel: w84 -> [w86]
            tunnel: [w85] -> w83
            stop <- w89 stop-if-true
            n43 = call <vilib>:"WPI_CANTalonSRX_GetStatus.vi"("CAN Talon SRX Ref"=w86) -> ("Talon SRX Status"=w92:T15, "CAN Talon SRX Ref"=w91:T7)  [unwired: 8 in, 1 out]
            n44 = Unbundle By Name(w92) -> ("Encoder Position"=w88:dbl)
            "Encoder Position" <- w88
            n45 = Greater?(x=-20000.0 ("y"), y=w88) -> (0:w89:bool)
            n46 = case shown="False" w89 {
              tunnel: [0.1 ("x") 0.0 ("x")] -> w90
              frame False {
              }
              frame True {
              }
            }
            n47 = call <vilib>:"WPI_MotorControlSetOutput.vi"("Output"=w90, "MotorControlDevRef"=w91) -> ("MotorControlDevRef"=w85:T7)  [unwired: 7 in, 2 out]
          }
        }
        frame #4 {
          w97 = T14 77 items=["Slot 0 - P"=1, "Slot 0 - I"=2, "Slot 0 - D"=3, "Slot 0 - F"=4, "Slot 0 - I Zone"=5, "Slot 0 - Ramp Rate"=6, "Slot 1 - P"=11, "Slot 1 - I"=12, "Slot 1 - D"=13, "Slot 1 - F"=14, "Slot 1 - I Zone"=15, "Slot 1 - Ramp Rate"=16, "Soft Limit - Forward"=21, "Soft Limit - Reverse"=22, "Soft Limit - Forward Enable"=23, "Soft Limit - Reverse Enable"=24, "On Boot - Brake Mode"=31, "On Boot - Limit Normally Closed - Forward"=32, "On Boot - Limit Normally Closed - Reverse"=33, "On Boot - Limit Disabled - Forward"=34, "On Boot - Limit Disabled - Reverse"=35, "Fault - Over Temp"=41, "Fault - Under Voltage"=42, "Fault - Forward Limit"=43, "Fault - Reverse Limit"=44, "Fault - Hardware Failure"=45, "Fault - Forward Soft Limit"=46, "Fault - Reverse Soft Limit"=47, "Sticky Fault - Over Temp"=48, "Sticky Fault - Under Voltage"=49, "Sticky Fault - Forward Limit"=50, "Sticky Fault - Reverse Limit"=51, "Sticky Fault - Forward Soft Limit"=52, "Sticky Fault - Reverse Soft Limit"=53, "Applied Throttle"=61, "Closed-Loop Error"=62, "Select Feedback Device"=63, "Reverse Closed-Loop Output"=64, "Mode Select"=65, "Profile Slot Select"=66, "Ramp Throttle"=67, "Reverse Feedback Sensor"=68, "Limit Switch Enabled"=69, "Limit Switch Closed - Forward"=70, "Limit Switch Closed - Reverse"=71, "Sensor Position"=73, "Sensor Velocity"=74, "Current"=75, "Brake is Enabled"=76, "Encoder Position"=77, "Encoder Velocity"=78, "Encoder Index Rise Events"=79, "Encoder A Pin State"=80, "Encoder B Pin State"=81, "Encoder Index Pin State"=82, "Analog In with Overflow"=83, "Analog In Velocity"=84, "Temperature"=85, "Battery Voltage"=86, "Reset Count"=87, "Reset Flags"=88, "Firmware Version"=89, "Settings Changed"=90, "Quad Filter Enable"=91, "Ignore Disable Broadcast"=92, "I Accumulator"=93, "Status 1 Frame Rate Ms"=94, "Status 2 Frame Rate Ms"=95, "Status 3 Frame Rate Ms"=96, "Status 4 Frame Rate Ms"=97, "Status 6 Frame Rate Ms"=98, "Status 7 Frame Rate Ms"=99, "Enable Index Pin Clear Position"=100, "Peak Positive Output"=104, "Nominal Positive Output"=105, "Peak Negative Output"=106, "Nominal Negative Output"=107, "Quad Index Pin Polarity"=108, "Status 8 Frame Rate Ms"=109, "Allow Position Overflow"=110, "Slot 0 - Allowable Closed-Loop Error"=111, "Number Potentiometer Turns"=112, "Encoder Codes Per Rev"=113, "Pulse Width Decoded Position"=114, "Analog Position"=115, "Voltage Compensation Rate (V/s)"=116, "Slot 1 - Allowable Closed-Loop Error"=117, "Motion Profile Has Underrun Err"=119, "Reserved 120"=120, "Legacy Control Mode"=121, "Motion Magic Acceleration"=122, "Motion Magic Cruise Velocity"=123, "Status 10 Frame Rate"=124, "Current Limit Threshold"=125, "CustomParam0"=137, "CustomParam1"=138, "PersStorageSaving"=139, "ClearPositionOnLimitF"=144, "ClearPositionOnLimitR"=145, "NominalBatteryVoltage"=146, "SampleVelocityPeriod"=147, "SampleVelocityWindow"=148] ("Parameter")
          n48 = Unbundle By Name(w95) -> ("CAN.Device Number"=w98:u8)
          n49 = call <vilib>:"WPI_CANTalonSRX_SetParameter.vi"("Value"=0.0, "Parameter"=w97, "Device ID (0)"=w98) -> ()  [unwired: 7 in, 2 out]
        }
        frame #5 {
          n50 = while {
            tunnel: w100 -> [w102]
            tunnel: [w101] -> w99
            stop <- w105 stop-if-true
            n51 = call <vilib>:"WPI_CANTalonSRX_GetStatus.vi"("CAN Talon SRX Ref"=w102) -> ("Talon SRX Status"=w108:T15, "CAN Talon SRX Ref"=w107:T7)  [unwired: 8 in, 1 out]
            n52 = Unbundle By Name(w108) -> ("Encoder Position"=w104:dbl)
            "Encoder Position 3" <- w104
            n53 = Less?(x=500000.0, y=w104) -> (x < y?=w105:bool)
            n54 = case shown="False" w105 {
              tunnel: [-0.5 ("x") 0.0 ("x")] -> w106
              frame False {
              }
              frame True {
              }
            }
            n55 = call <vilib>:"WPI_MotorControlSetOutput.vi"("Output"=w106, "MotorControlDevRef"=w107) -> ("MotorControlDevRef"=w101:T7)  [unwired: 7 in, 2 out]
          }
        }
        frame #6 {
          w113 = T14 77 items=["Slot 0 - P"=1, "Slot 0 - I"=2, "Slot 0 - D"=3, "Slot 0 - F"=4, "Slot 0 - I Zone"=5, "Slot 0 - Ramp Rate"=6, "Slot 1 - P"=11, "Slot 1 - I"=12, "Slot 1 - D"=13, "Slot 1 - F"=14, "Slot 1 - I Zone"=15, "Slot 1 - Ramp Rate"=16, "Soft Limit - Forward"=21, "Soft Limit - Reverse"=22, "Soft Limit - Forward Enable"=23, "Soft Limit - Reverse Enable"=24, "On Boot - Brake Mode"=31, "On Boot - Limit Normally Closed - Forward"=32, "On Boot - Limit Normally Closed - Reverse"=33, "On Boot - Limit Disabled - Forward"=34, "On Boot - Limit Disabled - Reverse"=35, "Fault - Over Temp"=41, "Fault - Under Voltage"=42, "Fault - Forward Limit"=43, "Fault - Reverse Limit"=44, "Fault - Hardware Failure"=45, "Fault - Forward Soft Limit"=46, "Fault - Reverse Soft Limit"=47, "Sticky Fault - Over Temp"=48, "Sticky Fault - Under Voltage"=49, "Sticky Fault - Forward Limit"=50, "Sticky Fault - Reverse Limit"=51, "Sticky Fault - Forward Soft Limit"=52, "Sticky Fault - Reverse Soft Limit"=53, "Applied Throttle"=61, "Closed-Loop Error"=62, "Select Feedback Device"=63, "Reverse Closed-Loop Output"=64, "Mode Select"=65, "Profile Slot Select"=66, "Ramp Throttle"=67, "Reverse Feedback Sensor"=68, "Limit Switch Enabled"=69, "Limit Switch Closed - Forward"=70, "Limit Switch Closed - Reverse"=71, "Sensor Position"=73, "Sensor Velocity"=74, "Current"=75, "Brake is Enabled"=76, "Encoder Position"=77, "Encoder Velocity"=78, "Encoder Index Rise Events"=79, "Encoder A Pin State"=80, "Encoder B Pin State"=81, "Encoder Index Pin State"=82, "Analog In with Overflow"=83, "Analog In Velocity"=84, "Temperature"=85, "Battery Voltage"=86, "Reset Count"=87, "Reset Flags"=88, "Firmware Version"=89, "Settings Changed"=90, "Quad Filter Enable"=91, "Ignore Disable Broadcast"=92, "I Accumulator"=93, "Status 1 Frame Rate Ms"=94, "Status 2 Frame Rate Ms"=95, "Status 3 Frame Rate Ms"=96, "Status 4 Frame Rate Ms"=97, "Status 6 Frame Rate Ms"=98, "Status 7 Frame Rate Ms"=99, "Enable Index Pin Clear Position"=100, "Peak Positive Output"=104, "Nominal Positive Output"=105, "Peak Negative Output"=106, "Nominal Negative Output"=107, "Quad Index Pin Polarity"=108, "Status 8 Frame Rate Ms"=109, "Allow Position Overflow"=110, "Slot 0 - Allowable Closed-Loop Error"=111, "Number Potentiometer Turns"=112, "Encoder Codes Per Rev"=113, "Pulse Width Decoded Position"=114, "Analog Position"=115, "Voltage Compensation Rate (V/s)"=116, "Slot 1 - Allowable Closed-Loop Error"=117, "Motion Profile Has Underrun Err"=119, "Reserved 120"=120, "Legacy Control Mode"=121, "Motion Magic Acceleration"=122, "Motion Magic Cruise Velocity"=123, "Status 10 Frame Rate"=124, "Current Limit Threshold"=125, "CustomParam0"=137, "CustomParam1"=138, "PersStorageSaving"=139, "ClearPositionOnLimitF"=144, "ClearPositionOnLimitR"=145, "NominalBatteryVoltage"=146, "SampleVelocityPeriod"=147, "SampleVelocityWindow"=148] ("Parameter")
          n56 = Unbundle By Name(w111) -> ("CAN.Device Number"=w112:u8)
          n57 = call <vilib>:"WPI_CANTalonSRX_SetParameter.vi"("Value"=0.0, "Parameter"=w113, "Device ID (0)"=w112) -> ()  [unwired: 7 in, 2 out]
        }
        frame #7 {
          n58 = while {
            tunnel: w116 -> [w118]
            tunnel: [w117] -> w115
            stop <- w121 stop-if-true
            n59 = call <vilib>:"WPI_CANTalonSRX_GetStatus.vi"("CAN Talon SRX Ref"=w118) -> ("Talon SRX Status"=w124:T15, "CAN Talon SRX Ref"=w123:T7)  [unwired: 8 in, 1 out]
            n60 = Unbundle By Name(w124) -> ("Encoder Position"=w120:dbl)
            "Encoder Position 4" <- w120
            n61 = Greater?(x=-20000.0, y=w120) -> (0:w121:bool)
            n62 = case shown="False" w121 {
              tunnel: [0.3 ("x") 0.0 ("x")] -> w122
              frame False {
              }
              frame True {
              }
            }
            n63 = call <vilib>:"WPI_MotorControlSetOutput.vi"("Output"=w122, "MotorControlDevRef"=w123) -> ("MotorControlDevRef"=w117:T7)  [unwired: 7 in, 2 out]
          }
        }
        frame #8 {
          w129 = T14 77 items=["Slot 0 - P"=1, "Slot 0 - I"=2, "Slot 0 - D"=3, "Slot 0 - F"=4, "Slot 0 - I Zone"=5, "Slot 0 - Ramp Rate"=6, "Slot 1 - P"=11, "Slot 1 - I"=12, "Slot 1 - D"=13, "Slot 1 - F"=14, "Slot 1 - I Zone"=15, "Slot 1 - Ramp Rate"=16, "Soft Limit - Forward"=21, "Soft Limit - Reverse"=22, "Soft Limit - Forward Enable"=23, "Soft Limit - Reverse Enable"=24, "On Boot - Brake Mode"=31, "On Boot - Limit Normally Closed - Forward"=32, "On Boot - Limit Normally Closed - Reverse"=33, "On Boot - Limit Disabled - Forward"=34, "On Boot - Limit Disabled - Reverse"=35, "Fault - Over Temp"=41, "Fault - Under Voltage"=42, "Fault - Forward Limit"=43, "Fault - Reverse Limit"=44, "Fault - Hardware Failure"=45, "Fault - Forward Soft Limit"=46, "Fault - Reverse Soft Limit"=47, "Sticky Fault - Over Temp"=48, "Sticky Fault - Under Voltage"=49, "Sticky Fault - Forward Limit"=50, "Sticky Fault - Reverse Limit"=51, "Sticky Fault - Forward Soft Limit"=52, "Sticky Fault - Reverse Soft Limit"=53, "Applied Throttle"=61, "Closed-Loop Error"=62, "Select Feedback Device"=63, "Reverse Closed-Loop Output"=64, "Mode Select"=65, "Profile Slot Select"=66, "Ramp Throttle"=67, "Reverse Feedback Sensor"=68, "Limit Switch Enabled"=69, "Limit Switch Closed - Forward"=70, "Limit Switch Closed - Reverse"=71, "Sensor Position"=73, "Sensor Velocity"=74, "Current"=75, "Brake is Enabled"=76, "Encoder Position"=77, "Encoder Velocity"=78, "Encoder Index Rise Events"=79, "Encoder A Pin State"=80, "Encoder B Pin State"=81, "Encoder Index Pin State"=82, "Analog In with Overflow"=83, "Analog In Velocity"=84, "Temperature"=85, "Battery Voltage"=86, "Reset Count"=87, "Reset Flags"=88, "Firmware Version"=89, "Settings Changed"=90, "Quad Filter Enable"=91, "Ignore Disable Broadcast"=92, "I Accumulator"=93, "Status 1 Frame Rate Ms"=94, "Status 2 Frame Rate Ms"=95, "Status 3 Frame Rate Ms"=96, "Status 4 Frame Rate Ms"=97, "Status 6 Frame Rate Ms"=98, "Status 7 Frame Rate Ms"=99, "Enable Index Pin Clear Position"=100, "Peak Positive Output"=104, "Nominal Positive Output"=105, "Peak Negative Output"=106, "Nominal Negative Output"=107, "Quad Index Pin Polarity"=108, "Status 8 Frame Rate Ms"=109, "Allow Position Overflow"=110, "Slot 0 - Allowable Closed-Loop Error"=111, "Number Potentiometer Turns"=112, "Encoder Codes Per Rev"=113, "Pulse Width Decoded Position"=114, "Analog Position"=115, "Voltage Compensation Rate (V/s)"=116, "Slot 1 - Allowable Closed-Loop Error"=117, "Motion Profile Has Underrun Err"=119, "Reserved 120"=120, "Legacy Control Mode"=121, "Motion Magic Acceleration"=122, "Motion Magic Cruise Velocity"=123, "Status 10 Frame Rate"=124, "Current Limit Threshold"=125, "CustomParam0"=137, "CustomParam1"=138, "PersStorageSaving"=139, "ClearPositionOnLimitF"=144, "ClearPositionOnLimitR"=145, "NominalBatteryVoltage"=146, "SampleVelocityPeriod"=147, "SampleVelocityWindow"=148] ("Parameter")
          n64 = Unbundle By Name(w127) -> ("CAN.Device Number"=w128:u8)
          n65 = call <vilib>:"WPI_CANTalonSRX_SetParameter.vi"("Value"=0.0, "Parameter"=w129, "Device ID (0)"=w128) -> ()  [unwired: 7 in, 2 out]
        }
      }
    }
    frame "SHOOT" {
      n66 = call-poly <vilib>:"WPI_RobotDriveArcadeDrive.vi"("error in (no error)"=w155, "Y axis value"=0.0, "X axis value"=0.0, "RobotDriveDevRef"=w156) -> ("error out"=w152:errorcluster, "RobotDriveDevRef"=w153:T11)  [unwired: 5 in, 1 out]
      n67 = call <vilib>:"WPI_RobotDriveDelayAndUpdateSafety.vi"("error in (no error)"=w152, "Delay (s)"=2.0, "RobotDriveDevRef"=w153) -> ("error out"=w148:errorcluster, "RobotDriveDevRef 2"=w149:T11)  [unwired: 7 in]
      n68 = call-poly <vilib>:"WPI_RobotDriveArcadeDrive.vi"("error in (no error)"=w148, "Y axis value"=0.85, "RobotDriveDevRef"=w149) -> ("error out"=w145:errorcluster, "RobotDriveDevRef"=w146:T11)  [unwired: 6 in, 1 out]
      n69 = call <vilib>:"WPI_RobotDriveDelayAndUpdateSafety.vi"("error in (no error)"=w145, "Delay (s)"=1.25, "RobotDriveDevRef"=w146) -> ("error out"=w134:errorcluster, "RobotDriveDevRef 2"=w135:T11)  [unwired: 7 in]
      n70 = call-poly <vilib>:"WPI_RobotDriveArcadeDrive.vi"("error in (no error)"=w134, "Y axis value"=0.0, "RobotDriveDevRef"=w135) -> ("error out"=w137:errorcluster, "RobotDriveDevRef"=w136:T11)  [unwired: 6 in, 1 out]
      n71 = call <vilib>:"WPI_RobotDriveDelayAndUpdateSafety.vi"("error in (no error)"=w137, "Delay (s)"=0.1, "RobotDriveDevRef"=w136) -> ("error out"=w132:errorcluster, "RobotDriveDevRef 2"=w131:T11)  [unwired: 7 in]
      n72 = Merge Errors(w143, w142) -> (w141:errorcluster)
      n73 = Merge Errors(w132, w141) -> (w140:errorcluster)
      n74 = call <vilib>:"WPI_CANTalonSRX_SetReference.vi"("error in (no error)"=w140, "Feedback Reference"=WPI_CANTalonSRX_APIFeedbackSelect."CTR Magnetic Enc (Relative)", "CAN Talon SRX Ref"=w186) -> ("error out"=w185:errorcluster, "CAN Talon SRX Ref"=w194:T7)  [unwired: 7 in]
      n75 = call <vilib>:"WPI_MotorControlSetOutput.vi"("error in (no error)"=w140, "Output"=0.75, "MotorControlDevRef"=w173) -> ("error out"=w170:errorcluster, "MotorControlDevRef"=w168:T7)  [unwired: 6 in, 1 out]
      n76 = call <vilib>:"WPI_CANTalonSRX_SetPID.vi"("CAN Talon SRX Ref"=w194, "P"=0.0, "I"=0.0, "D"=0.0, "error in (no error)"=w185, "F"=0.01, "I Zone"=0.0, "Ramp Rate"=0.0) -> ("CAN Talon SRX Ref"=w191:T7, "error out"=w184:errorcluster)  [unwired: 6 in]
      n77 = call <vilib>:"WPI_CANTalonSRX_ChangeMode.vi"("error in (no error)"=w184, "Output"=9800.0 ("y"), "Control Mode"=WPI_CANTalonSRX_APIControlMode."Speed", "CAN Talon SRX Ref"=w191) -> ("error out"=w183:errorcluster, "CAN Talon SRX Ref"=w187:T7)  [unwired: 6 in]
      n78 = call <vilib>:"WPI_CANTalonSRX_GetStatus.vi"("error in (no error)"=w183, "CAN Talon SRX Ref"=w187) -> ("error out"=w171:errorcluster)  [unwired: 7 in, 2 out]
      n79 = Merge Errors(w171, w170) -> (w169:errorcluster)
      n80 = call <vilib>:"WPI_RobotDriveDelayAndUpdateSafety.vi"("error in (no error)"=w169, "Delay (s)"=9.0, "RobotDriveDevRef"=w131) -> ("error out"=w167:errorcluster, "RobotDriveDevRef 2"=w182:T11)  [unwired: 7 in]
      n81 = call <vilib>:"WPI_MotorControlSetOutput.vi"("error in (no error)"=w167, "Output"=0.0, "MotorControlDevRef"=w168) -> ("error out"=w139:errorcluster)  [unwired: 6 in, 2 out]
      n82 = call-poly <vilib>:"WPI_RobotDriveArcadeDrive.vi"("error in (no error)"=w139, "Y axis value"=0.0, "X axis value"=0.4, "RobotDriveDevRef"=w182) -> ("error out"=w179:errorcluster, "RobotDriveDevRef"=w180:T11)  [unwired: 5 in, 1 out]
      n83 = call <vilib>:"WPI_RobotDriveDelayAndUpdateSafety.vi"("error in (no error)"=w179, "Delay (s)"=1.0, "RobotDriveDevRef"=w180) -> ("error out"=w160:errorcluster, "RobotDriveDevRef 2"=w159:T11)  [unwired: 7 in]
      n84 = call-poly <vilib>:"WPI_RobotDriveArcadeDrive.vi"("error in (no error)"=w160, "Y axis value"=-0.8, "X axis value"=0.0, "RobotDriveDevRef"=w159) -> ("error out"=w163:errorcluster, "RobotDriveDevRef"=w164:T11)  [unwired: 5 in, 1 out]
      n85 = call <vilib>:"WPI_RobotDriveDelayAndUpdateSafety.vi"("error in (no error)"=w163, "Delay (s)"=2.25, "RobotDriveDevRef"=w164) -> ("error out"=w157:errorcluster, "RobotDriveDevRef 2"=w158:T11)  [unwired: 7 in]
      n86 = call-poly <vilib>:"WPI_RobotDriveArcadeDrive.vi"("error in (no error)"=w157, "Y axis value"=0.0, "X axis value"=0.0, "RobotDriveDevRef"=w158) -> ()  [unwired: 5 in, 3 out]
    }
    frame "SHOOT2" {
      n87 = call-poly <vilib>:"WPI_RobotDriveArcadeDrive.vi"("error in (no error)"=w225, "Y axis value"=0.0, "X axis value"=0.0, "RobotDriveDevRef"=w224) -> ("error out"=w223:errorcluster, "RobotDriveDevRef"=w222:T11)  [unwired: 5 in, 1 out]
      n88 = call <vilib>:"WPI_RobotDriveDelayAndUpdateSafety.vi"("error in (no error)"=w223, "Delay (s)"=2.0, "RobotDriveDevRef"=w222) -> ("error out"=w218:errorcluster, "RobotDriveDevRef 2"=w217:T11)  [unwired: 7 in]
      n89 = call-poly <vilib>:"WPI_RobotDriveArcadeDrive.vi"("error in (no error)"=w218, "Y axis value"=0.5, "RobotDriveDevRef"=w217) -> ("error out"=w214:errorcluster, "RobotDriveDevRef"=w215:T11)  [unwired: 6 in, 1 out]
      n90 = call <vilib>:"WPI_RobotDriveDelayAndUpdateSafety.vi"("error in (no error)"=w214, "Delay (s)"=1.0, "RobotDriveDevRef"=w215) -> ("error out"=w212:errorcluster, "RobotDriveDevRef 2"=w211:T11)  [unwired: 7 in]
      n91 = call-poly <vilib>:"WPI_RobotDriveArcadeDrive.vi"("error in (no error)"=w212, "Y axis value"=0.0, "RobotDriveDevRef"=w211) -> ("error out"=w209:errorcluster, "RobotDriveDevRef"=w210:T11)  [unwired: 6 in, 1 out]
      n92 = Merge Errors(w203, w202) -> (w201:errorcluster)
      n93 = call <vilib>:"WPI_RobotDriveDelayAndUpdateSafety.vi"("error in (no error)"=w209, "Delay (s)"=0.1, "RobotDriveDevRef"=w210) -> ("error out"=w200:errorcluster, "RobotDriveDevRef 2"=w206:T11)  [unwired: 7 in]
      n94 = Merge Errors(w200, w201) -> (w199:errorcluster)
      n95 = call <vilib>:"WPI_CANTalonSRX_SetReference.vi"("error in (no error)"=w199, "Feedback Reference"=WPI_CANTalonSRX_APIFeedbackSelect."CTR Magnetic Enc (Relative)", "CAN Talon SRX Ref"=w205) -> ("error out"=w274:errorcluster, "CAN Talon SRX Ref"=w282:T7)  [unwired: 7 in]
      n96 = call <vilib>:"WPI_MotorControlSetOutput.vi"("error in (no error)"=w199, "Output"=0.75, "MotorControlDevRef"=w204) -> ("error out"=w262:errorcluster, "MotorControlDevRef"=w260:T7)  [unwired: 6 in, 1 out]
      n97 = call <vilib>:"WPI_CANTalonSRX_SetPID.vi"("CAN Talon SRX Ref"=w282, "P"=0.0, "I"=0.0, "D"=0.0, "error in (no error)"=w274, "F"=0.01, "I Zone"=0.0, "Ramp Rate"=0.0) -> ("CAN Talon SRX Ref"=w279:T7, "error out"=w273:errorcluster)  [unwired: 6 in]
      n98 = call <vilib>:"WPI_CANTalonSRX_ChangeMode.vi"("error in (no error)"=w273, "Output"=9800.0 ("y"), "Control Mode"=WPI_CANTalonSRX_APIControlMode."Speed", "CAN Talon SRX Ref"=w279) -> ("error out"=w272:errorcluster, "CAN Talon SRX Ref"=w275:T7)  [unwired: 6 in]
      n99 = call <vilib>:"WPI_CANTalonSRX_GetStatus.vi"("error in (no error)"=w272, "CAN Talon SRX Ref"=w275) -> ("error out"=w263:errorcluster, "CAN Talon SRX Ref"=w245:T7)  [unwired: 7 in, 1 out]
      n100 = Merge Errors(w263, w262) -> (w261:errorcluster)
      n101 = call <vilib>:"WPI_RobotDriveDelayAndUpdateSafety.vi"("error in (no error)"=w261, "Delay (s)"=9.0, "RobotDriveDevRef"=w206) -> ("error out"=w244:errorcluster, "RobotDriveDevRef 2"=w271:T11)  [unwired: 7 in]
      n102 = call <vilib>:"WPI_CANTalonSRX_ChangeMode.vi"("error in (no error)"=w244, "Output"=0.0 ("y"), "Control Mode"=WPI_CANTalonSRX_APIControlMode."Speed", "CAN Talon SRX Ref"=w245) -> ("error out"=w246:errorcluster, "CAN Talon SRX Ref"=w247:T7)  [unwired: 6 in]
      n103 = call <vilib>:"WPI_MotorControlSetOutput.vi"("error in (no error)"=w244, "Output"=0.0, "MotorControlDevRef"=w260) -> ("error out"=w242:errorcluster)  [unwired: 6 in, 2 out]
      n104 = call <vilib>:"WPI_CANTalonSRX_GetStatus.vi"("error in (no error)"=w246, "CAN Talon SRX Ref"=w247) -> ("error out"=w243:errorcluster)  [unwired: 7 in, 2 out]
      n105 = Merge Errors(w243, w242) -> (w241:errorcluster)
      n106 = call <vilib>:"WPI_RobotDriveTankDrive.vi"("error in (no error)"=w241, "Right axis value"=0.6 ("Y axis value"), "Left axis value"=0.6, "RobotDriveDevRef"=w271) -> ("error out"=w269:errorcluster, "RobotDriveDevRef"=w270:T11)  [unwired: 5 in, 1 out]
      n107 = call <vilib>:"WPI_RobotDriveDelayAndUpdateSafety.vi"("error in (no error)"=w269, "Delay (s)"=0.25, "RobotDriveDevRef"=w270) -> ("error out"=w253:errorcluster, "RobotDriveDevRef 2"=w252:T11)  [unwired: 7 in]
      n108 = call-poly <vilib>:"WPI_RobotDriveArcadeDrive.vi"("error in (no error)"=w253, "Y axis value"=0.0, "X axis value"=-0.8, "RobotDriveDevRef"=w252) -> ("error out"=w256:errorcluster, "RobotDriveDevRef"=w257:T11)  [unwired: 5 in, 1 out]
      n109 = call <vilib>:"WPI_RobotDriveDelayAndUpdateSafety.vi"("error in (no error)"=w256, "Delay (s)"=0.5, "RobotDriveDevRef"=w257) -> ("error out"=w250:errorcluster, "RobotDriveDevRef 2"=w251:T11)  [unwired: 7 in]
      n110 = call-poly <vilib>:"WPI_RobotDriveArcadeDrive.vi"("error in (no error)"=w250, "Y axis value"=-0.5, "X axis value"=-0.55, "RobotDriveDevRef"=w251) -> ("error out"=w239:errorcluster, "RobotDriveDevRef"=w240:T11)  [unwired: 5 in, 1 out]
      n111 = call <vilib>:"WPI_RobotDriveDelayAndUpdateSafety.vi"("error in (no error)"=w239, "Delay (s)"=1.0, "RobotDriveDevRef"=w240) -> ("error out"=w237:errorcluster, "RobotDriveDevRef 2"=w236:T11)  [unwired: 7 in]
      n112 = call-poly <vilib>:"WPI_RobotDriveArcadeDrive.vi"("error in (no error)"=w237, "Y axis value"=-0.5 ("X axis value"), "RobotDriveDevRef"=w236) -> ("error out"=w231:errorcluster, "RobotDriveDevRef"=w232:T11)  [unwired: 6 in, 1 out]
      n113 = call <vilib>:"WPI_RobotDriveDelayAndUpdateSafety.vi"("error in (no error)"=w231, "Delay (s)"=2.0, "RobotDriveDevRef"=w232) -> ("error out"=w228:errorcluster, "RobotDriveDevRef 2"=w229:T11)  [unwired: 7 in]
      n114 = call-poly <vilib>:"WPI_RobotDriveArcadeDrive.vi"("error in (no error)"=w228, "Y axis value"=0.0, "X axis value"=0.0, "RobotDriveDevRef"=w229) -> ()  [unwired: 5 in, 3 out]
    }
    frame "SHOOTBLUE" {
      n115 = call <vilib>:"WPI_CANTalonSRX_SetReference.vi"("error in (no error)"=w288, "Feedback Reference"=WPI_CANTalonSRX_APIFeedbackSelect."CTR Magnetic Enc (Relative)", "CAN Talon SRX Ref"=w287) -> ("error out"=w320:errorcluster, "CAN Talon SRX Ref"=w328:T7)  [unwired: 7 in]
      n116 = call <vilib>:"WPI_MotorControlSetOutput.vi"("error in (no error)"=w289, "Output"=0.75, "MotorControlDevRef"=w290) -> ("error out"=w306:errorcluster, "MotorControlDevRef"=w304:T7)  [unwired: 6 in, 1 out]
      n117 = call <vilib>:"WPI_CANTalonSRX_SetPID.vi"("CAN Talon SRX Ref"=w328, "P"=0.0, "I"=0.0, "D"=0.0, "error in (no error)"=w320, "F"=0.01, "I Zone"=0.0, "Ramp Rate"=0.0) -> ("CAN Talon SRX Ref"=w325:T7, "error out"=w319:errorcluster)  [unwired: 6 in]
      n118 = call <vilib>:"WPI_CANTalonSRX_ChangeMode.vi"("error in (no error)"=w319, "Output"=9800.0 ("y"), "Control Mode"=WPI_CANTalonSRX_APIControlMode."Speed", "CAN Talon SRX Ref"=w325) -> ("error out"=w318:errorcluster, "CAN Talon SRX Ref"=w321:T7)  [unwired: 6 in]
      n119 = call <vilib>:"WPI_CANTalonSRX_GetStatus.vi"("error in (no error)"=w318, "CAN Talon SRX Ref"=w321) -> ("error out"=w307:errorcluster)  [unwired: 7 in, 2 out]
      n120 = Merge Errors(w307, w306) -> (w305:errorcluster)
      n121 = call <vilib>:"WPI_RobotDriveDelayAndUpdateSafety.vi"("error in (no error)"=w305, "Delay (s)"=10.0, "RobotDriveDevRef"=w291) -> ("error out"=w303:errorcluster, "RobotDriveDevRef 2"=w317:T11)  [unwired: 7 in]
      n122 = call <vilib>:"WPI_MotorControlSetOutput.vi"("error in (no error)"=w303, "Output"=0.0, "MotorControlDevRef"=w304) -> ("error out"=w292:errorcluster)  [unwired: 6 in, 2 out]
      n123 = call-poly <vilib>:"WPI_RobotDriveArcadeDrive.vi"("error in (no error)"=w292, "Y axis value"=0.0, "X axis value"=0.4, "RobotDriveDevRef"=w317) -> ("error out"=w314:errorcluster, "RobotDriveDevRef"=w315:T11)  [unwired: 5 in, 1 out]
      n124 = call <vilib>:"WPI_RobotDriveDelayAndUpdateSafety.vi"("error in (no error)"=w314, "Delay (s)"=1.0, "RobotDriveDevRef"=w315) -> ("error out"=w296:errorcluster, "RobotDriveDevRef 2"=w295:T11)  [unwired: 7 in]
      n125 = call-poly <vilib>:"WPI_RobotDriveArcadeDrive.vi"("error in (no error)"=w296, "Y axis value"=-0.6, "X axis value"=0.0, "RobotDriveDevRef"=w295) -> ("error out"=w299:errorcluster, "RobotDriveDevRef"=w300:T11)  [unwired: 5 in, 1 out]
      n126 = call <vilib>:"WPI_RobotDriveDelayAndUpdateSafety.vi"("error in (no error)"=w299, "Delay (s)"=3.0, "RobotDriveDevRef"=w300) -> ("error out"=w293:errorcluster, "RobotDriveDevRef 2"=w294:T11)  [unwired: 7 in]
      n127 = call-poly <vilib>:"WPI_RobotDriveArcadeDrive.vi"("error in (no error)"=w293, "Y axis value"=0.0, "X axis value"=0.0, "RobotDriveDevRef"=w294) -> ()  [unwired: 5 in, 3 out]
    }
    frame "SHOOTRED" {
      # "SHOOTRED"
      n128 = call <vilib>:"WPI_CANTalonSRX_SetReference.vi"("error in (no error)"=w385, "Feedback Reference"=WPI_CANTalonSRX_APIFeedbackSelect."CTR Magnetic Enc (Relative)", "CAN Talon SRX Ref"=w386) -> ("error out"=w384:errorcluster, "CAN Talon SRX Ref"=w394:T7)  [unwired: 7 in]
      n129 = call <vilib>:"WPI_MotorControlSetOutput.vi"("error in (no error)"=w372, "Output"=0.75, "MotorControlDevRef"=w373) -> ("error out"=w369:errorcluster, "MotorControlDevRef"=w367:T7)  [unwired: 6 in, 1 out]
      n130 = call <vilib>:"WPI_CANTalonSRX_SetPID.vi"("CAN Talon SRX Ref"=w394, "P"=0.0, "I"=0.0, "D"=0.0, "error in (no error)"=w384, "F"=0.01, "I Zone"=0.0, "Ramp Rate"=0.0) -> ("CAN Talon SRX Ref"=w391:T7, "error out"=w383:errorcluster)  [unwired: 6 in]
      n131 = call <vilib>:"WPI_CANTalonSRX_ChangeMode.vi"("error in (no error)"=w383, "Output"=9800.0 ("y"), "Control Mode"=WPI_CANTalonSRX_APIControlMode."Speed", "CAN Talon SRX Ref"=w391) -> ("error out"=w382:errorcluster, "CAN Talon SRX Ref"=w387:T7)  [unwired: 6 in]
      n132 = call <vilib>:"WPI_CANTalonSRX_GetStatus.vi"("error in (no error)"=w382, "CAN Talon SRX Ref"=w387) -> ("error out"=w370:errorcluster, "CAN Talon SRX Ref"=w352:T7)  [unwired: 7 in, 1 out]
      n133 = Merge Errors(w370, w369) -> (w368:errorcluster)
      n134 = call <vilib>:"WPI_RobotDriveDelayAndUpdateSafety.vi"("error in (no error)"=w368, "Delay (s)"=10.0, "RobotDriveDevRef"=w380) -> ("error out"=w351:errorcluster, "RobotDriveDevRef 2"=w381:T11)  [unwired: 7 in]
      n135 = call <vilib>:"WPI_CANTalonSRX_ChangeMode.vi"("error in (no error)"=w351, "Output"=0.0 ("y"), "Control Mode"=WPI_CANTalonSRX_APIControlMode."Speed", "CAN Talon SRX Ref"=w352) -> ("error out"=w353:errorcluster, "CAN Talon SRX Ref"=w354:T7)  [unwired: 6 in]
      n136 = call <vilib>:"WPI_MotorControlSetOutput.vi"("error in (no error)"=w351, "Output"=0.0, "MotorControlDevRef"=w367) -> ("error out"=w349:errorcluster)  [unwired: 6 in, 2 out]
      n137 = call <vilib>:"WPI_CANTalonSRX_GetStatus.vi"("error in (no error)"=w353, "CAN Talon SRX Ref"=w354) -> ("error out"=w350:errorcluster)  [unwired: 7 in, 2 out]
      n138 = Merge Errors(w350, w349) -> (w348:errorcluster)
      n139 = call <vilib>:"WPI_RobotDriveTankDrive.vi"("error in (no error)"=w348, "Right axis value"=0.6 ("Y axis value"), "Left axis value"=0.6, "RobotDriveDevRef"=w381) -> ("error out"=w378:errorcluster, "RobotDriveDevRef"=w379:T11)  [unwired: 5 in, 1 out]
      n140 = call <vilib>:"WPI_RobotDriveDelayAndUpdateSafety.vi"("error in (no error)"=w378, "Delay (s)"=0.25, "RobotDriveDevRef"=w379) -> ("error out"=w360:errorcluster, "RobotDriveDevRef 2"=w359:T11)  [unwired: 7 in]
      n141 = call-poly <vilib>:"WPI_RobotDriveArcadeDrive.vi"("error in (no error)"=w360, "Y axis value"=0.0, "X axis value"=-0.8, "RobotDriveDevRef"=w359) -> ("error out"=w363:errorcluster, "RobotDriveDevRef"=w364:T11)  [unwired: 5 in, 1 out]
      n142 = call <vilib>:"WPI_RobotDriveDelayAndUpdateSafety.vi"("error in (no error)"=w363, "Delay (s)"=0.5, "RobotDriveDevRef"=w364) -> ("error out"=w357:errorcluster, "RobotDriveDevRef 2"=w358:T11)  [unwired: 7 in]
      n143 = call-poly <vilib>:"WPI_RobotDriveArcadeDrive.vi"("error in (no error)"=w357, "Y axis value"=-0.5, "X axis value"=-0.55, "RobotDriveDevRef"=w358) -> ("error out"=w346:errorcluster, "RobotDriveDevRef"=w347:T11)  [unwired: 5 in, 1 out]
      n144 = call <vilib>:"WPI_RobotDriveDelayAndUpdateSafety.vi"("error in (no error)"=w346, "Delay (s)"=1.0, "RobotDriveDevRef"=w347) -> ("error out"=w344:errorcluster, "RobotDriveDevRef 2"=w343:T11)  [unwired: 7 in]
      n145 = call-poly <vilib>:"WPI_RobotDriveArcadeDrive.vi"("error in (no error)"=w344, "Y axis value"=-0.5 ("X axis value"), "RobotDriveDevRef"=w343) -> ("error out"=w338:errorcluster, "RobotDriveDevRef"=w339:T11)  [unwired: 6 in, 1 out]
      n146 = call <vilib>:"WPI_RobotDriveDelayAndUpdateSafety.vi"("error in (no error)"=w338, "Delay (s)"=2.0, "RobotDriveDevRef"=w339) -> ("error out"=w335:errorcluster, "RobotDriveDevRef 2"=w336:T11)  [unwired: 7 in]
      n147 = call-poly <vilib>:"WPI_RobotDriveArcadeDrive.vi"("error in (no error)"=w335, "Y axis value"=0.0, "X axis value"=0.0, "RobotDriveDevRef"=w336) -> ()  [unwired: 5 in, 3 out]
    }
    frame "NEW" {
      n148 = while {
        tunnel: w420 -> [w512]
        tunnel: w419 -> [w511]
        tunnel: [w505] -> w421
        tunnel: [w504] -> w422
        tunnel: w418 -> [w503]
        tunnel: w417 -> [w497]
        tunnel: [w493] -> w416
        tunnel: [w492] -> w415
        tunnel: w406 -> [w491]
        tunnel: [w491] -> w405
        stop <- w494 stop-if-true
        n149 = call <vilib>:"WPI_EncoderGet.vi"("EncoderDevRef"=w503) -> ("Distance"=w502:dbl, "EncoderDevRef"=w493:T3)  [unwired: 5 in, 4 out]
        n150 = call <vilib>:"WPI_EncoderGet.vi"("EncoderDevRef"=w512) -> ("Distance"=w510:dbl, "EncoderDevRef"=w504:T3)  [unwired: 5 in, 4 out]
        n151 = Greater?(x=w502, y=4.0) -> (0:w495:bool)
        n152 = Greater?(x=w510, y=4.0) -> (0:w496:bool)
        n153 = Select(t=0.0, s=w495, f=-0.3) -> (s? t:f=w498:dbl)
        n154 = Select(t=0.0, s=w496, f=-0.3) -> (s? t:f=w506:dbl)
        n155 = And(x=w496, y=w495) -> (x .and. y?=w494:bool)
        n156 = call <vilib>:"WPI_MotorControlSetOutput.vi"("Output"=w498, "MotorControlDevRef"=w497) -> ("MotorControlDevRef"=w492:T7)  [unwired: 7 in, 2 out]
        n157 = call <vilib>:"WPI_MotorControlSetOutput.vi"("Output"=w506, "MotorControlDevRef"=w511) -> ("MotorControlDevRef"=w505:T7)  [unwired: 7 in, 2 out]
      }
      n158 = while {
        tunnel: [w487] -> w414
        tunnel: [w486] -> w413
        tunnel: w422 -> [w485]
        tunnel: w421 -> [w484]
        tunnel: w416 -> [w480]
        tunnel: w415 -> [w479]
        tunnel: [w480] -> w412
        tunnel: [w479] -> w411
        tunnel: w405 -> [w478]
        tunnel: [w478] -> w404
        stop <- w481 continue-if-true
        n159 = call <vilib>:"WPI_EncoderGet.vi"("EncoderDevRef"=w485) -> ("Distance"=w483:dbl, "EncoderDevRef"=w487:T3)  [unwired: 5 in, 4 out]
        n160 = Greater?(x=4.0 ("y"), y=w483) -> (0:w481:bool)
        n161 = Select(t=0.3, s=w481, f=0.0 ("Output")) -> (s? t:f=w488:dbl)
        n162 = call <vilib>:"WPI_MotorControlSetOutput.vi"("Output"=w488, "MotorControlDevRef"=w484) -> ("MotorControlDevRef"=w486:T7)  [unwired: 7 in, 2 out]
      }
      n163 = while {
        tunnel: w414 -> [w477]
        tunnel: w413 -> [w476]
        tunnel: [w470] -> w407
        tunnel: [w469] -> w408
        tunnel: w412 -> [w468]
        tunnel: w411 -> [w462]
        tunnel: [w458] -> w409
        tunnel: [w457] -> w410
        tunnel: w404 -> [w456]
        tunnel: [w456] -> w403
        stop <- w459 stop-if-true
        n164 = call <vilib>:"WPI_EncoderGet.vi"("EncoderDevRef"=w468) -> ("Distance"=w467:dbl, "EncoderDevRef"=w458:T3)  [unwired: 5 in, 4 out]
        n165 = call <vilib>:"WPI_EncoderGet.vi"("EncoderDevRef"=w477) -> ("Distance"=w475:dbl, "EncoderDevRef"=w469:T3)  [unwired: 5 in, 4 out]
        n166 = Greater?(x=w467, y=4.0) -> (0:w460:bool)
        n167 = Greater?(x=w475, y=4.0) -> (0:w461:bool)
        n168 = Select(t=0.0, s=w460, f=-0.3) -> (s? t:f=w463:dbl)
        n169 = Select(t=0.0, s=w461, f=-0.3) -> (s? t:f=w471:dbl)
        n170 = And(x=w461, y=w460) -> (x .and. y?=w459:bool)
        n171 = call <vilib>:"WPI_MotorControlSetOutput.vi"("Output"=w463, "MotorControlDevRef"=w462) -> ("MotorControlDevRef"=w457:T7)  [unwired: 7 in, 2 out]
        n172 = call <vilib>:"WPI_MotorControlSetOutput.vi"("Output"=w471, "MotorControlDevRef"=w476) -> ("MotorControlDevRef"=w470:T7)  [unwired: 7 in, 2 out]
      }
      n173 = while {
        tunnel: w410 -> [w447]
        tunnel: w409 -> [w446]
        tunnel: w408 -> [w444]
        tunnel: w407 -> [w445]
        tunnel: w403 -> [w455]
        tunnel: [w447] -> w402
        tunnel: [w446] -> w401
        tunnel: [w445] -> w400
        tunnel: [w444] -> w399
        stop <- w448 stop-if-true
        n174 = global read "Robot Global Data.vi" "LOWER LIMIT"() -> (w451:bool)
        n175 = Select(t=0.0, s=w451, f=-0.5) -> (s? t:f=w452:dbl)
        n176 = call <vilib>:"WPI_MotorControlSetOutput.vi"("Output"=w452, "MotorControlDevRef"=w455) -> ("Motor Output"=w450:dbl)  [unwired: 7 in, 2 out]
        n177 = Equal?(x=w450, y=0.0) -> (x = y?=w448:bool)
      }
      n178 = while {
        tunnel: [w438] -> _
        tunnel: [w437] -> _
        tunnel: [w428] -> _
        tunnel: [w427] -> _
        tunnel: w402 -> [w426]
        tunnel: w401 -> [w425]
        tunnel: w400 -> [w424]
        tunnel: w399 -> [w423]
        stop <- w429 stop-if-true
        n179 = call <vilib>:"WPI_EncoderGet.vi"("EncoderDevRef"=w425) -> ("Distance"=w436:dbl, "EncoderDevRef"=w428:T3)  [unwired: 5 in, 4 out]
        n180 = call <vilib>:"WPI_EncoderGet.vi"("EncoderDevRef"=w423) -> ("Distance"=w443:dbl, "EncoderDevRef"=w437:T3)  [unwired: 5 in, 4 out]
        n181 = Greater?(x=w436, y=0.0) -> (0:w430:bool)
        n182 = Greater?(x=w443, y=0.0) -> (0:w431:bool)
        n183 = Select(t=-0.3, s=w430, f=0.0) -> (s? t:f=w432:dbl)
        n184 = Select(t=-0.3, s=w431, f=0.0) -> (s? t:f=w439:dbl)
        n185 = And(x=w431, y=w430) -> (x .and. y?=w429:bool)
        n186 = call <vilib>:"WPI_MotorControlSetOutput.vi"("Output"=w432, "MotorControlDevRef"=w426) -> ("MotorControlDevRef"=w427:T7)  [unwired: 7 in, 2 out]
        n187 = call <vilib>:"WPI_MotorControlSetOutput.vi"("Output"=w439, "MotorControlDevRef"=w424) -> ("MotorControlDevRef"=w438:T7)  [unwired: 7 in, 2 out]
      }
    }
    frame "GEAR1" {
      n188 = while {
        tunnel: w531 -> [w612]
        tunnel: w532 -> [w592]
        tunnel: [w608] -> w527
        tunnel: [w607] -> w522
        tunnel: w530 -> [w599]
        tunnel: w529 -> [w596]
        tunnel: [w599] -> w520
        tunnel: [w603] -> w526
        tunnel: w528 -> [w602]
        tunnel: [w602] -> w524
        stop <- w597 continue-if-true
        n189 = call <vilib>:"WPI_CANTalonSRX_GetStatus.vi"("CAN Talon SRX Ref"=w592) -> ("Talon SRX Status"=w590:T15, "CAN Talon SRX Ref"=w591:T7)  [unwired: 8 in, 1 out]
        n190 = call <vilib>:"WPI_CANTalonSRX_GetStatus.vi"("CAN Talon SRX Ref"=w596) -> ("Talon SRX Status"=w594:T15, "CAN Talon SRX Ref"=w595:T7)  [unwired: 8 in, 1 out]
        n191 = Unbundle By Name(w594) -> ("Current"=→"CURRENT":dbl)
        n192 = call <vilib>:"WPI_EncoderGet.vi"("EncoderDevRef"=w612) -> ("Distance"=w598:dbl, "EncoderDevRef"=w607:T3)  [unwired: 5 in, 4 out]
        "Distance" <- w598
        n193 = Unbundle By Name(w590) -> ("Current"=→"Current":dbl)
        n194 = In Range and Coerce(upper limit=15.9, x=w598, lower limit=0.0) -> (In Range?=w597:bool)  [unwired: 1 out]
        n195 = Select(t=0.3, s=w597, f=0.0) -> (s? t:f=w604:dbl)
        n196 = Select(t=0.3, s=w597, f=0.0) -> (s? t:f=w609:dbl)
        n197 = call <vilib>:"WPI_MotorControlSetOutput.vi"("Output"=w604, "MotorControlDevRef"=w595) -> ("MotorControlDevRef"=w603:T7)  [unwired: 7 in, 2 out]
        n198 = call <vilib>:"WPI_MotorControlSetOutput.vi"("Output"=w609, "MotorControlDevRef"=w591) -> ("MotorControlDevRef"=w608:T7)  [unwired: 7 in, 2 out]
      }
      n199 = call <vilib>:"WPI_EncoderReset.vi"("EncoderDevRef"=w522) -> ("EncoderDevRef"=w521:T3)  [unwired: 9 in, 1 out]
      n200 = while {
        tunnel: [w568] -> w525
        tunnel: [w567] -> w519
        tunnel: [w563] -> w516
        tunnel: w521 -> [w559]
        tunnel: w527 -> [w558]
        tunnel: w526 -> [w557]
        tunnel: [w556] -> w523
        tunnel: w524 -> [w556]
        tunnel: w520 -> [w555]
        stop <- w549 continue-if-true
        n201 = call <vilib>:"WPI_EncoderGet.vi"("EncoderDevRef"=w555) -> ("Distance"=w554:dbl)  [unwired: 5 in, 5 out]
        n202 = call <vilib>:"WPI_EncoderGet.vi"("EncoderDevRef"=w559) -> ("Distance"=w560:dbl, "EncoderDevRef"=w567:T3)  [unwired: 5 in, 4 out]
        n203 = In Range and Coerce(upper limit=0.4, x=w554, lower limit=0.0) -> (In Range?=w551:bool)  [unwired: 1 out]
        n204 = In Range and Coerce(upper limit=5.9, x=w560, lower limit=0.0) -> (In Range?=w550:bool)  [unwired: 1 out]
        n205 = Select(t=0.3, s=w551, f=0.0) -> (s? t:f=w564:dbl)
        n206 = Select(t=-0.3, s=w550, f=0.0) -> (s? t:f=w569:dbl)
        n207 = And(x=w551, y=w550) -> (x .and. y?=w549:bool)
        n208 = call <vilib>:"WPI_MotorControlSetOutput.vi"("Output"=w564, "MotorControlDevRef"=w557) -> ("MotorControlDevRef"=w563:T7)  [unwired: 7 in, 2 out]
        n209 = call <vilib>:"WPI_MotorControlSetOutput.vi"("Output"=w569, "MotorControlDevRef"=w558) -> ("MotorControlDevRef"=w568:T7)  [unwired: 7 in, 2 out]
      }
      n210 = call <vilib>:"WPI_EncoderReset.vi"("EncoderDevRef"=w519) -> ("EncoderDevRef"=w518:T3)  [unwired: 9 in, 1 out]
      n211 = while {
        tunnel: [w585] -> w515
        tunnel: [w584] -> w514
        tunnel: [w580] -> w513
        tunnel: w525 -> [w575]
        tunnel: w516 -> [w574]
        tunnel: w523 -> [w572]
        tunnel: w518 -> [w573]
        tunnel: [w572] -> _
        stop <- w576 continue-if-true
        n212 = call <vilib>:"WPI_EncoderGet.vi"("EncoderDevRef"=w573) -> ("Distance"=w577:dbl, "EncoderDevRef"=w584:T3)  [unwired: 5 in, 4 out]
        n213 = In Range and Coerce(upper limit=5.0, x=w577, lower limit=0.0) -> (In Range?=w576:bool)  [unwired: 1 out]
        n214 = Select(t=-0.3, s=w576, f=0.0) -> (s? t:f=w581:dbl)
        n215 = Select(t=-0.3, s=w576, f=0.0) -> (s? t:f=w586:dbl)
        n216 = call <vilib>:"WPI_MotorControlSetOutput.vi"("Output"=w581, "MotorControlDevRef"=w574) -> ("MotorControlDevRef"=w580:T7)  [unwired: 7 in, 2 out]
        n217 = call <vilib>:"WPI_MotorControlSetOutput.vi"("Output"=w586, "MotorControlDevRef"=w575) -> ("MotorControlDevRef"=w585:T7)  [unwired: 7 in, 2 out]
      }
      n218 = call <vilib>:"WPI_EncoderReset.vi"("EncoderDevRef"=w514) -> ("EncoderDevRef"=w517:T3)  [unwired: 9 in, 1 out]
      n219 = while {
        tunnel: [w545] -> _
        tunnel: [w544] -> _
        tunnel: [w540] -> _
        tunnel: w515 -> [w535]
        tunnel: w513 -> [w534]
        tunnel: w517 -> [w533]
        stop <- w536 continue-if-true
        n220 = call <vilib>:"WPI_EncoderGet.vi"("EncoderDevRef"=w533) -> ("Distance"=w537:dbl, "EncoderDevRef"=w544:T3)  [unwired: 5 in, 4 out]
        n221 = In Range and Coerce(upper limit=5.0, x=w537, lower limit=0.0) -> (In Range?=w536:bool)  [unwired: 1 out]
        n222 = Select(t=0.4, s=w536, f=0.0) -> (s? t:f=w541:dbl)
        n223 = Select(t=0.4, s=w536, f=0.0) -> (s? t:f=w546:dbl)
        n224 = call <vilib>:"WPI_MotorControlSetOutput.vi"("Output"=w541, "MotorControlDevRef"=w534) -> ("MotorControlDevRef"=w540:T7)  [unwired: 7 in, 2 out]
        n225 = call <vilib>:"WPI_MotorControlSetOutput.vi"("Output"=w546, "MotorControlDevRef"=w535) -> ("MotorControlDevRef"=w545:T7)  [unwired: 7 in, 2 out]
      }
    }
    frame "CENTERGEAR" {
      n226 = call-poly <vilib>:"WPI_RobotDriveArcadeDrive.vi"("error in (no error)"=w635, "Y axis value"=0.5, "RobotDriveDevRef"=w636) -> ("error out"=w632:errorcluster, "RobotDriveDevRef"=w633:T11)  [unwired: 6 in, 1 out]
      n227 = call <vilib>:"WPI_RobotDriveDelayAndUpdateSafety.vi"("error in (no error)"=w632, "Delay (s)"=3.0, "RobotDriveDevRef"=w633) -> ("error out"=w629:errorcluster, "RobotDriveDevRef 2"=w627:T11)  [unwired: 7 in]
      n228 = call <vilib>:"WPI_MotorControlSetOutput.vi"("error in (no error)"=w629, "Output"=-0.6, "MotorControlDevRef"=w630) -> ("error out"=w626:errorcluster)  [unwired: 6 in, 2 out]
      n229 = call <vilib>:"WPI_RobotDriveDelayAndUpdateSafety.vi"("error in (no error)"=w626, "Delay (s)"=2.0, "RobotDriveDevRef"=w627) -> ("error out"=w622:errorcluster, "RobotDriveDevRef 2"=w624:T11)  [unwired: 7 in]
      n230 = call-poly <vilib>:"WPI_RobotDriveArcadeDrive.vi"("error in (no error)"=w622, "Y axis value"=-0.4, "RobotDriveDevRef"=w624) -> ("error out"=w621:errorcluster, "RobotDriveDevRef"=w620:T11)  [unwired: 6 in, 1 out]
      n231 = call <vilib>:"WPI_RobotDriveDelayAndUpdateSafety.vi"("error in (no error)"=w621, "Delay (s)"=2.0, "RobotDriveDevRef"=w620) -> ("error out"=w617:errorcluster, "RobotDriveDevRef 2"=w618:T11)  [unwired: 7 in]
      n232 = call-poly <vilib>:"WPI_RobotDriveArcadeDrive.vi"("error in (no error)"=w617, "Y axis value"=0.0, "RobotDriveDevRef"=w618) -> ("error out"=w614:errorcluster, "RobotDriveDevRef"=w615:T11)  [unwired: 6 in, 1 out]
      n233 = call <vilib>:"WPI_RobotDriveDelayAndUpdateSafety.vi"("error in (no error)"=w614, "Delay (s)"=1.0, "RobotDriveDevRef"=w615) -> ()  [unwired: 7 in, 2 out]
    }
    frame "ENCODER" {
      n234 = while {
        tunnel: w650 -> [w705]
        tunnel: w649 -> [w703]
        tunnel: w648 -> [w704]
        tunnel: w647 -> [w702]
        tunnel: w646 -> [w684]
        tunnel: [w688] -> w645
        tunnel: [w687] -> w644
        tunnel: [w686] -> w643
        tunnel: [w685] -> w642
        tunnel: [w684] -> w641
        stop <- w689 continue-if-true
        n235 = call <vilib>:"WPI_EncoderGet.vi"("EncoderDevRef"=w704) -> ("Distance"=w695:dbl, "EncoderDevRef"=w685:T3)  [unwired: 5 in, 4 out]
        n236 = call <vilib>:"WPI_EncoderGet.vi"("EncoderDevRef"=w705) -> ("Distance"=w701:dbl, "EncoderDevRef"=w687:T3)  [unwired: 5 in, 4 out]
        n237 = Less?(x=w701, y=78.0) -> (x < y?=w691:bool)
        n238 = Less?(x=w695, y=78.0) -> (x < y?=w690:bool)
        n239 = Select(t=0.3, s=w691, f=0.0) -> (s? t:f=w697:dbl)
        n240 = Select(t=0.3, s=w690, f=0.0) -> (s? t:f=w693:dbl)
        n241 = And(x=w691, y=w690) -> (x .and. y?=w689:bool)
        n242 = call <vilib>:"WPI_MotorControlSetOutput.vi"("Output"=w697, "MotorControlDevRef"=w703) -> ("MotorControlDevRef"=w686:T7)  [unwired: 7 in, 2 out]
        n243 = call <vilib>:"WPI_MotorControlSetOutput.vi"("Output"=w693, "MotorControlDevRef"=w702) -> ("MotorControlDevRef"=w688:T7)  [unwired: 7 in, 2 out]
      }
      n244 = while {
        tunnel: w645 -> [w681]
        tunnel: w644 -> [w678]
        tunnel: w643 -> [w679]
        tunnel: w642 -> [w680]
        tunnel: w641 -> [w683]
        tunnel: [w681] -> w639
        tunnel: [w680] -> w637
        tunnel: [w679] -> w640
        tunnel: [w678] -> w638
        stop <- w677 stop-if-true
        n245 = Wait (ms)(milliseconds to wait=u32 3000) -> (millisecond timer value=w676:u32)
        n246 = call <vilib>:"WPI_MotorControlSetOutput.vi"("Output"=-0.6, "MotorControlDevRef"=w683) -> ()  [unwired: 7 in, 3 out]
        n247 = Equal?(x=w676, y=u32 3000) -> (x = y?=w677:bool)
      }
      n248 = flat-sequence {
        tunnel: w637 -> [w651]
        frame #0 {
          n249 = call <vilib>:"WPI_EncoderReset.vi"("EncoderDevRef"=w651) -> ()  [unwired: 9 in, 2 out]
        }
      }
      n250 = flat-sequence {
        tunnel: w638 -> [w652]
        frame #0 {
          n251 = call <vilib>:"WPI_EncoderReset.vi"("EncoderDevRef"=w652) -> ()  [unwired: 9 in, 2 out]
        }
      }
      n252 = while {
        tunnel: w638 -> [w673]
        tunnel: w640 -> [w672]
        tunnel: w639 -> [w671]
        tunnel: [w657] -> _
        tunnel: [w656] -> _
        tunnel: [w655] -> _
        tunnel: [w654] -> _
        tunnel: w637 -> [w653]
        stop <- w658 continue-if-true
        n253 = call <vilib>:"WPI_EncoderGet.vi"("EncoderDevRef"=w653) -> ("Distance"=w664:dbl, "EncoderDevRef"=w654:T3)  [unwired: 5 in, 4 out]
        n254 = call <vilib>:"WPI_EncoderGet.vi"("EncoderDevRef"=w673) -> ("Distance"=w670:dbl, "EncoderDevRef"=w656:T3)  [unwired: 5 in, 4 out]
        n255 = Less?(x=w670, y=-40.0) -> (x < y?=w660:bool)
        n256 = Less?(x=w664, y=-40.0) -> (x < y?=w659:bool)
        n257 = Select(t=-0.3, s=w660, f=0.0) -> (s? t:f=w666:dbl)
        n258 = Select(t=-0.3, s=w659, f=0.0) -> (s? t:f=w662:dbl)
        n259 = And(x=w660, y=w659) -> (x .and. y?=w658:bool)
        n260 = call <vilib>:"WPI_MotorControlSetOutput.vi"("Output"=w666, "MotorControlDevRef"=w672) -> ("MotorControlDevRef"=w655:T7)  [unwired: 7 in, 2 out]
        n261 = call <vilib>:"WPI_MotorControlSetOutput.vi"("Output"=w662, "MotorControlDevRef"=w671) -> ("MotorControlDevRef"=w657:T7)  [unwired: 7 in, 2 out]
      }
    }
    frame "AUTO CENTER" {
      n262 = while {
        tunnel: w719 -> [w774]
        tunnel: w718 -> [w773]
        tunnel: [w767] -> w710
        tunnel: [w766] -> w709
        tunnel: w717 -> [w765]
        tunnel: w716 -> [w759]
        tunnel: [w755] -> w708
        tunnel: [w754] -> w707
        tunnel: w715 -> [w753]
        tunnel: [w753] -> w706
        stop <- w756 stop-if-true
        n263 = call <vilib>:"WPI_EncoderGet.vi"("EncoderDevRef"=w765) -> ("Distance"=w764:dbl, "EncoderDevRef"=w755:T3)  [unwired: 5 in, 4 out]
        n264 = call <vilib>:"WPI_EncoderGet.vi"("EncoderDevRef"=w774) -> ("Distance"=w772:dbl, "EncoderDevRef"=w766:T3)  [unwired: 5 in, 4 out]
        n265 = Greater?(x=w764, y=4.0) -> (0:w757:bool)
        n266 = Greater?(x=w772, y=4.0) -> (0:w758:bool)
        n267 = Select(t=0.0, s=w757, f=-0.3) -> (s? t:f=w760:dbl)
        n268 = Select(t=0.0, s=w758, f=-0.3) -> (s? t:f=w768:dbl)
        n269 = And(x=w758, y=w757) -> (x .and. y?=w756:bool)
        n270 = call <vilib>:"WPI_MotorControlSetOutput.vi"("Output"=w760, "MotorControlDevRef"=w759) -> ("MotorControlDevRef"=w754:T7)  [unwired: 7 in, 2 out]
        n271 = call <vilib>:"WPI_MotorControlSetOutput.vi"("Output"=w768, "MotorControlDevRef"=w773) -> ("MotorControlDevRef"=w767:T7)  [unwired: 7 in, 2 out]
      }
      n272 = while {
        tunnel: w707 -> [w744]
        tunnel: w708 -> [w743]
        tunnel: w709 -> [w741]
        tunnel: w710 -> [w742]
        tunnel: w706 -> [w752]
        tunnel: [w744] -> w711
        tunnel: [w743] -> w712
        tunnel: [w742] -> w713
        tunnel: [w741] -> w714
        stop <- w745 stop-if-true
        n273 = global read "Robot Global Data.vi" "LOWER LIMIT"() -> (w748:bool)
        n274 = Select(t=0.0, s=w748, f=-0.5) -> (s? t:f=w749:dbl)
        n275 = call <vilib>:"WPI_MotorControlSetOutput.vi"("Output"=w749, "MotorControlDevRef"=w752) -> ("Motor Output"=w747:dbl)  [unwired: 7 in, 2 out]
        n276 = Equal?(x=w747, y=0.0) -> (x = y?=w745:bool)
      }
      n277 = while {
        tunnel: [w735] -> _
        tunnel: [w734] -> _
        tunnel: [w725] -> _
        tunnel: [w724] -> _
        tunnel: w711 -> [w723]
        tunnel: w712 -> [w722]
        tunnel: w713 -> [w721]
        tunnel: w714 -> [w720]
        stop <- w726 stop-if-true
        n278 = call <vilib>:"WPI_EncoderGet.vi"("EncoderDevRef"=w722) -> ("Distance"=w733:dbl, "EncoderDevRef"=w725:T3)  [unwired: 5 in, 4 out]
        n279 = call <vilib>:"WPI_EncoderGet.vi"("EncoderDevRef"=w720) -> ("Distance"=w740:dbl, "EncoderDevRef"=w734:T3)  [unwired: 5 in, 4 out]
        n280 = Greater?(x=w733, y=0.0) -> (0:w727:bool)
        n281 = Greater?(x=w740, y=0.0) -> (0:w728:bool)
        n282 = Select(t=-0.3, s=w727, f=0.0) -> (s? t:f=w729:dbl)
        n283 = Select(t=-0.3, s=w728, f=0.0) -> (s? t:f=w736:dbl)
        n284 = And(x=w728, y=w727) -> (x .and. y?=w726:bool)
        n285 = call <vilib>:"WPI_MotorControlSetOutput.vi"("Output"=w729, "MotorControlDevRef"=w723) -> ("MotorControlDevRef"=w724:T7)  [unwired: 7 in, 2 out]
        n286 = call <vilib>:"WPI_MotorControlSetOutput.vi"("Output"=w736, "MotorControlDevRef"=w721) -> ("MotorControlDevRef"=w735:T7)  [unwired: 7 in, 2 out]
      }
    }
    frame "AUTO LEFT NS" {
      n287 = while {
        tunnel: w795 -> [w852]
        tunnel: [w848] -> w792
        tunnel: [w847] -> w777
        tunnel: w794 -> [w843]
        tunnel: [w842] -> w791
        tunnel: w793 -> [w841]
        tunnel: [w841] -> w790
        tunnel: w775 -> [w836]
        stop <- w837 continue-if-true
        n288 = call <vilib>:"WPI_EncoderGet.vi"("EncoderDevRef"=w836) -> ("Distance"=w838:dbl, "EncoderDevRef"=w847:T3)  [unwired: 5 in, 4 out]
        "Distance 3" <- w838
        n289 = In Range and Coerce(upper limit=12.0, x=w838, lower limit=0.0) -> (In Range?=w837:bool)  [unwired: 1 out]
        n290 = Select(t=0.35, s=w837, f=0.0) -> (s? t:f=w844:dbl)
        n291 = Select(t=0.35, s=w837, f=0.0) -> (s? t:f=w849:dbl)
        n292 = call <vilib>:"WPI_MotorControlSetOutput.vi"("Output"=w844, "MotorControlDevRef"=w843) -> ("MotorControlDevRef"=w842:T7)  [unwired: 7 in, 2 out]
        n293 = call <vilib>:"WPI_MotorControlSetOutput.vi"("Output"=w849, "MotorControlDevRef"=w852) -> ("MotorControlDevRef"=w848:T7)  [unwired: 7 in, 2 out]
      }
      n294 = while {
        tunnel: w777 -> [w835]
        tunnel: w792 -> [w834]
        tunnel: [w830] -> w789
        tunnel: [w829] -> w776
        tunnel: w791 -> [w825]
        tunnel: [w824] -> w788
        tunnel: w790 -> [w823]
        tunnel: [w823] -> w787
        stop <- w819 continue-if-true
        n295 = call <vilib>:"WPI_EncoderGet.vi"("EncoderDevRef"=w835) -> ("Distance"=w820:dbl, "EncoderDevRef"=w829:T3)  [unwired: 5 in, 4 out]
        "Distance 4" <- w820
        n296 = In Range and Coerce(upper limit=2.4, x=w820, lower limit=0.0) -> (In Range?=w819:bool)  [unwired: 1 out]
        n297 = Select(t=0.0, s=w819, f=0.0) -> (s? t:f=w826:dbl)
        n298 = Select(t=0.35, s=w819, f=0.0) -> (s? t:f=w831:dbl)
        n299 = call <vilib>:"WPI_MotorControlSetOutput.vi"("Output"=w826, "MotorControlDevRef"=w825) -> ("MotorControlDevRef"=w824:T7)  [unwired: 7 in, 2 out]
        n300 = call <vilib>:"WPI_MotorControlSetOutput.vi"("Output"=w831, "MotorControlDevRef"=w834) -> ("MotorControlDevRef"=w830:T7)  [unwired: 7 in, 2 out]
      }
      n301 = flat-sequence {
        tunnel: w777 -> [w797]
        frame #0 {
          n302 = call <vilib>:"WPI_EncoderReset.vi"("EncoderDevRef"=w797) -> ()  [unwired: 9 in, 2 out]
        }
      }
      n303 = while {
        tunnel: w776 -> [w818]
        tunnel: w789 -> [w817]
        tunnel: [w813] -> w786
        tunnel: [w812] -> w785
        tunnel: w788 -> [w808]
        tunnel: [w807] -> w784
        tunnel: w787 -> [w806]
        tunnel: [w806] -> w783
        stop <- w802 continue-if-true
        n304 = call <vilib>:"WPI_EncoderGet.vi"("EncoderDevRef"=w818) -> ("Distance"=w803:dbl, "EncoderDevRef"=w812:T3)  [unwired: 5 in, 4 out]
        "Distance 5" <- w803
        n305 = In Range and Coerce(upper limit=4.0, x=w803, lower limit=0.0) -> (In Range?=w802:bool)  [unwired: 1 out]
        n306 = Select(t=0.35, s=w802, f=0.0) -> (s? t:f=w809:dbl)
        n307 = Select(t=0.35, s=w802, f=0.0) -> (s? t:f=w814:dbl)
        n308 = call <vilib>:"WPI_MotorControlSetOutput.vi"("Output"=w809, "MotorControlDevRef"=w808) -> ("MotorControlDevRef"=w807:T7)  [unwired: 7 in, 2 out]
        n309 = call <vilib>:"WPI_MotorControlSetOutput.vi"("Output"=w814, "MotorControlDevRef"=w817) -> ("MotorControlDevRef"=w813:T7)  [unwired: 7 in, 2 out]
      }
      n310 = flat-sequence {
        tunnel: w776 -> [w796]
        frame #0 {
          n311 = call <vilib>:"WPI_EncoderReset.vi"("EncoderDevRef"=w796) -> ()  [unwired: 9 in, 2 out]
        }
      }
      n312 = while {
        tunnel: w784 -> [w859]
        tunnel: w785 -> [w857]
        tunnel: w786 -> [w858]
        tunnel: w783 -> [w860]
        tunnel: [w859] -> w780
        tunnel: [w858] -> w782
        tunnel: [w857] -> w781
        tunnel: [w856] -> w779
        tunnel: [w853] -> w778
        stop <- w855 stop-if-true
        n313 = call <vilib>:"WPI_MotorControlSetOutput.vi"("Output"=-0.5 ("f"), "MotorControlDevRef"=w860) -> ("error out"=w853:errorcluster, "MotorControlDevRef"=w856:T7)  [unwired: 7 in, 1 out]
        n314 = global read "Robot Global Data.vi" "LOWER LIMIT"() -> (w855:bool)
      }
      n315 = while {
        tunnel: w782 -> [_]
        tunnel: w781 -> [_]
        tunnel: w780 -> [_]
        tunnel: w779 -> [w800]
        tunnel: w778 -> [w799]
        stop <- FALSE stop-if-true
        n316 = call <vilib>:"WPI_MotorControlSetOutput.vi"("error in (no error)"=w799, "Output"=0.0, "MotorControlDevRef"=w800) -> ()  [unwired: 6 in, 3 out]
      }
    }
    frame "MIDDLE" {
      n317 = call-poly <vilib>:"WPI_RobotDriveArcadeDrive.vi"("error in (no error)"=w890, "Y axis value"=0.45, "RobotDriveDevRef"=w891) -> ("error out"=w887:errorcluster, "RobotDriveDevRef"=w888:T11)  [unwired: 6 in, 1 out]
      n318 = call <vilib>:"WPI_RobotDriveDelayAndUpdateSafety.vi"("error in (no error)"=w887, "Delay (s)"=2.0, "RobotDriveDevRef"=w888) -> ("error out"=w885:errorcluster, "RobotDriveDevRef 2"=w884:T11)  [unwired: 7 in]
      n319 = call-poly <vilib>:"WPI_RobotDriveArcadeDrive.vi"("error in (no error)"=w885, "Y axis value"=0.0, "RobotDriveDevRef"=w884) -> ("error out"=w881:errorcluster, "RobotDriveDevRef"=w882:T11)  [unwired: 6 in, 1 out]
      n320 = call <vilib>:"WPI_RobotDriveDelayAndUpdateSafety.vi"("error in (no error)"=w881, "Delay (s)"=0.5, "RobotDriveDevRef"=w882) -> ("error out"=w879:errorcluster, "RobotDriveDevRef 2"=w877:T11)  [unwired: 7 in]
      n321 = call <vilib>:"WPI_MotorControlSetOutput.vi"("error in (no error)"=w879, "Output"=-0.7, "MotorControlDevRef"=w878) -> ("error out"=w876:errorcluster, "MotorControlDevRef"=w872:T7)  [unwired: 6 in, 1 out]
      n322 = call <vilib>:"WPI_RobotDriveDelayAndUpdateSafety.vi"("error in (no error)"=w876, "Delay (s)"=1.5, "RobotDriveDevRef"=w877) -> ("error out"=w873:errorcluster, "RobotDriveDevRef 2"=w870:T11)  [unwired: 7 in]
      n323 = call <vilib>:"WPI_MotorControlSetOutput.vi"("error in (no error)"=w873, "Output"=0.0, "MotorControlDevRef"=w872) -> ("error out"=w869:errorcluster)  [unwired: 6 in, 2 out]
      n324 = call-poly <vilib>:"WPI_RobotDriveArcadeDrive.vi"("error in (no error)"=w869, "Y axis value"=-0.4, "RobotDriveDevRef"=w870) -> ("error out"=w866:errorcluster, "RobotDriveDevRef"=w867:T11)  [unwired: 6 in, 1 out]
      n325 = call <vilib>:"WPI_RobotDriveDelayAndUpdateSafety.vi"("error in (no error)"=w866, "Delay (s)"=2.0, "RobotDriveDevRef"=w867) -> ("error out"=w863:errorcluster, "RobotDriveDevRef 2"=w864:T11)  [unwired: 7 in]
      n326 = call-poly <vilib>:"WPI_RobotDriveArcadeDrive.vi"("error in (no error)"=w863, "Y axis value"=0.0, "X axis value"=0.0, "RobotDriveDevRef"=w864) -> ()  [unwired: 5 in, 3 out]
    }
    frame "RIGHTSIDE" {
      # "RIGHTSIDE"
      n327 = call-poly <vilib>:"WPI_RobotDriveArcadeDrive.vi"("error in (no error)"=w893, "Y axis value"=0.59, "RobotDriveDevRef"=w894) -> ("error out"=w933:errorcluster, "RobotDriveDevRef"=w934:T11)  [unwired: 6 in, 1 out]
      n328 = call <vilib>:"WPI_RobotDriveDelayAndUpdateSafety.vi"("error in (no error)"=w933, "Delay (s)"=1.8, "RobotDriveDevRef"=w934) -> ("error out"=w929:errorcluster, "RobotDriveDevRef 2"=w930:T11)  [unwired: 7 in]
      n329 = call-poly <vilib>:"WPI_RobotDriveArcadeDrive.vi"("error in (no error)"=w929, "X axis value"=0.36, "RobotDriveDevRef"=w930) -> ("error out"=w926:errorcluster, "RobotDriveDevRef"=w927:T11)  [unwired: 6 in, 1 out]
      n330 = call <vilib>:"WPI_RobotDriveDelayAndUpdateSafety.vi"("error in (no error)"=w926, "Delay (s)"=1.0, "RobotDriveDevRef"=w927) -> ("error out"=w923:errorcluster, "RobotDriveDevRef 2"=w924:T11)  [unwired: 7 in]
      n331 = call-poly <vilib>:"WPI_RobotDriveArcadeDrive.vi"("error in (no error)"=w923, "Y axis value"=0.5, "RobotDriveDevRef"=w924) -> ("error out"=w920:errorcluster, "RobotDriveDevRef"=w921:T11)  [unwired: 6 in, 1 out]
      n332 = call <vilib>:"WPI_RobotDriveDelayAndUpdateSafety.vi"("error in (no error)"=w920, "Delay (s)"=2.3, "RobotDriveDevRef"=w921) -> ("error out"=w917:errorcluster, "RobotDriveDevRef 2"=w918:T11)  [unwired: 7 in]
      n333 = call-poly <vilib>:"WPI_RobotDriveArcadeDrive.vi"("error in (no error)"=w917, "Y axis value"=0.0, "RobotDriveDevRef"=w918) -> ("error out"=w914:errorcluster, "RobotDriveDevRef"=w915:T11)  [unwired: 6 in, 1 out]
      n334 = call <vilib>:"WPI_RobotDriveDelayAndUpdateSafety.vi"("error in (no error)"=w914, "Delay (s)"=0.5, "RobotDriveDevRef"=w915) -> ("error out"=w912:errorcluster, "RobotDriveDevRef 2"=w910:T11)  [unwired: 7 in]
      n335 = call <vilib>:"WPI_MotorControlSetOutput.vi"("error in (no error)"=w912, "Output"=-0.7, "MotorControlDevRef"=w892) -> ("error out"=w909:errorcluster, "MotorControlDevRef"=w898:T7)  [unwired: 6 in, 1 out]
      n336 = call <vilib>:"WPI_RobotDriveDelayAndUpdateSafety.vi"("error in (no error)"=w909, "Delay (s)"=1.5, "RobotDriveDevRef"=w910) -> ("error out"=w897:errorcluster, "RobotDriveDevRef 2"=w907:T11)  [unwired: 7 in]
      n337 = call <vilib>:"WPI_MotorControlSetOutput.vi"("error in (no error)"=w897, "Output"=0.0, "MotorControlDevRef"=w898) -> ("error out"=w895:errorcluster)  [unwired: 6 in, 2 out]
      n338 = call-poly <vilib>:"WPI_RobotDriveArcadeDrive.vi"("error in (no error)"=w895, "Y axis value"=-0.4, "RobotDriveDevRef"=w907) -> ("error out"=w904:errorcluster, "RobotDriveDevRef"=w905:T11)  [unwired: 6 in, 1 out]
      n339 = call <vilib>:"WPI_RobotDriveDelayAndUpdateSafety.vi"("error in (no error)"=w904, "Delay (s)"=2.0, "RobotDriveDevRef"=w905) -> ("error out"=w902:errorcluster, "RobotDriveDevRef 2"=w901:T11)  [unwired: 7 in]
      n340 = call-poly <vilib>:"WPI_RobotDriveArcadeDrive.vi"("error in (no error)"=w902, "Y axis value"=0.0, "X axis value"=0.0, "RobotDriveDevRef"=w901) -> ()  [unwired: 5 in, 3 out]
    }
    frame "LEFTSIDE" {
      n341 = call-poly <vilib>:"WPI_RobotDriveArcadeDrive.vi"("error in (no error)"=w976, "Y axis value"=0.6, "RobotDriveDevRef"=w977) -> ("error out"=w974:errorcluster, "RobotDriveDevRef"=w975:T11)  [unwired: 6 in, 1 out]
      n342 = call <vilib>:"WPI_RobotDriveDelayAndUpdateSafety.vi"("error in (no error)"=w974, "Delay (s)"=2.0, "RobotDriveDevRef"=w975) -> ("error out"=w970:errorcluster, "RobotDriveDevRef 2"=w971:T11)  [unwired: 7 in]
      n343 = call-poly <vilib>:"WPI_RobotDriveArcadeDrive.vi"("error in (no error)"=w970, "X axis value"=-0.45, "RobotDriveDevRef"=w971) -> ("error out"=w967:errorcluster, "RobotDriveDevRef"=w968:T11)  [unwired: 6 in, 1 out]
      n344 = call <vilib>:"WPI_RobotDriveDelayAndUpdateSafety.vi"("error in (no error)"=w967, "Delay (s)"=1.0, "RobotDriveDevRef"=w968) -> ("error out"=w964:errorcluster, "RobotDriveDevRef 2"=w965:T11)  [unwired: 7 in]
      n345 = call-poly <vilib>:"WPI_RobotDriveArcadeDrive.vi"("error in (no error)"=w964, "Y axis value"=0.52, "RobotDriveDevRef"=w965) -> ("error out"=w961:errorcluster, "RobotDriveDevRef"=w962:T11)  [unwired: 6 in, 1 out]
      n346 = call <vilib>:"WPI_RobotDriveDelayAndUpdateSafety.vi"("error in (no error)"=w961, "Delay (s)"=2.25, "RobotDriveDevRef"=w962) -> ("error out"=w958:errorcluster, "RobotDriveDevRef 2"=w959:T11)  [unwired: 7 in]
      n347 = call-poly <vilib>:"WPI_RobotDriveArcadeDrive.vi"("error in (no error)"=w958, "Y axis value"=0.0, "RobotDriveDevRef"=w959) -> ("error out"=w955:errorcluster, "RobotDriveDevRef"=w956:T11)  [unwired: 6 in, 1 out]
      n348 = call <vilib>:"WPI_RobotDriveDelayAndUpdateSafety.vi"("error in (no error)"=w955, "Delay (s)"=0.5, "RobotDriveDevRef"=w956) -> ("error out"=w952:errorcluster, "RobotDriveDevRef 2"=w950:T11)  [unwired: 7 in]
      n349 = call <vilib>:"WPI_MotorControlSetOutput.vi"("error in (no error)"=w952, "Output"=-0.7, "MotorControlDevRef"=w953) -> ("error out"=w949:errorcluster, "MotorControlDevRef"=w938:T7)  [unwired: 6 in, 1 out]
      n350 = call <vilib>:"WPI_RobotDriveDelayAndUpdateSafety.vi"("error in (no error)"=w949, "Delay (s)"=1.5, "RobotDriveDevRef"=w950) -> ("error out"=w937:errorcluster, "RobotDriveDevRef 2"=w947:T11)  [unwired: 7 in]
      n351 = call <vilib>:"WPI_MotorControlSetOutput.vi"("error in (no error)"=w937, "Output"=0.0, "MotorControlDevRef"=w938) -> ("error out"=w935:errorcluster)  [unwired: 6 in, 2 out]
      n352 = call-poly <vilib>:"WPI_RobotDriveArcadeDrive.vi"("error in (no error)"=w935, "Y axis value"=-0.4, "RobotDriveDevRef"=w947) -> ("error out"=w944:errorcluster, "RobotDriveDevRef"=w945:T11)  [unwired: 6 in, 1 out]
      n353 = call <vilib>:"WPI_RobotDriveDelayAndUpdateSafety.vi"("error in (no error)"=w944, "Delay (s)"=2.0, "RobotDriveDevRef"=w945) -> ("error out"=w942:errorcluster, "RobotDriveDevRef 2"=w941:T11)  [unwired: 7 in]
      n354 = call-poly <vilib>:"WPI_RobotDriveArcadeDrive.vi"("error in (no error)"=w942, "Y axis value"=0.0, "X axis value"=0.0, "RobotDriveDevRef"=w941) -> ()  [unwired: 5 in, 3 out]
    }
    frame "Forward" {
      n355 = call-poly <vilib>:"WPI_RobotDriveArcadeDrive.vi"("error in (no error)"=w982, "Y axis value"=0.55, "RobotDriveDevRef"=w983) -> ("error out"=w978:errorcluster, "RobotDriveDevRef"=w980:T11)  [unwired: 6 in, 1 out]
      n356 = call <vilib>:"WPI_RobotDriveDelayAndUpdateSafety.vi"("error in (no error)"=w978, "Delay (s)"=2.8, "RobotDriveDevRef"=w980) -> ()  [unwired: 7 in, 2 out]
    }
    frame "GEAR DROP" {
      n357 = call-poly <vilib>:"WPI_RobotDriveArcadeDrive.vi"("error in (no error)"=w1007, "Y axis value"=0.45, "RobotDriveDevRef"=w1008) -> ("error out"=w1004:errorcluster, "RobotDriveDevRef"=w1005:T11)  [unwired: 6 in, 1 out]
      n358 = call <vilib>:"WPI_RobotDriveDelayAndUpdateSafety.vi"("error in (no error)"=w1004, "Delay (s)"=2.4, "RobotDriveDevRef"=w1005) -> ("error out"=w1002:errorcluster, "RobotDriveDevRef 2"=w1001:T11)  [unwired: 7 in]
      n359 = call-poly <vilib>:"WPI_RobotDriveArcadeDrive.vi"("error in (no error)"=w1002, "Y axis value"=0.0, "RobotDriveDevRef"=w1001) -> ("error out"=w998:errorcluster, "RobotDriveDevRef"=w999:T11)  [unwired: 6 in, 1 out]
      n360 = call <vilib>:"WPI_RobotDriveDelayAndUpdateSafety.vi"("error in (no error)"=w998, "Delay (s)"=0.5, "RobotDriveDevRef"=w999) -> ("error out"=w991:errorcluster, "RobotDriveDevRef 2"=w990:T11)  [unwired: 7 in]
      n361 = while {
        tunnel: w991 -> [w1020]
        tunnel: [w1017] -> w989
        tunnel: w988 -> [w1016]
        tunnel: [w1015] -> w987
        stop <- w1018 stop-if-true
        n362 = global read "Robot Global Data.vi" "LOWER LIMIT"() -> (w1018:bool)
        n363 = call <vilib>:"WPI_MotorControlSetOutput.vi"("error in (no error)"=w1020, "Output"=-0.6 ("f"), "MotorControlDevRef"=w1016) -> ("error out"=w1017:errorcluster, "MotorControlDevRef"=w1015:T7)  [unwired: 6 in, 1 out]
      }
      n364 = call-poly <vilib>:"WPI_RobotDriveArcadeDrive.vi"("error in (no error)"=w989, "Y axis value"=-0.4, "RobotDriveDevRef"=w990) -> ("error out"=w995:errorcluster, "RobotDriveDevRef"=w994:T11)  [unwired: 6 in, 1 out]
      n365 = call <vilib>:"WPI_RobotDriveDelayAndUpdateSafety.vi"("error in (no error)"=w995, "Delay (s)"=1.5, "RobotDriveDevRef"=w994) -> ("error out"=w986:errorcluster)  [unwired: 7 in, 1 out]
      n366 = while {
        tunnel: w987 -> [w1013]
        tunnel: w986 -> [w1011]
        tunnel: [w1010] -> w985
        tunnel: [w1009] -> w984
        stop <- w1014 stop-if-true
        n367 = call <vilib>:"WPI_MotorControlSetOutput.vi"("error in (no error)"=w1011, "Output"=0.6, "MotorControlDevRef"=w1013) -> ("error out"=w1009:errorcluster, "MotorControlDevRef"=w1010:T7)  [unwired: 6 in, 1 out]
        n368 = global read "Robot Global Data.vi" "UPPER LIMIT"() -> (w1014:bool)
      }
      n369 = call <vilib>:"WPI_MotorControlSetOutput.vi"("error in (no error)"=w984, "Output"=0.0, "MotorControlDevRef"=w985) -> ()  [unwired: 6 in, 3 out]
    }
  }
